vi "A170316-11_Auto.vi"() -> ()   [LabVIEW 2020]
uses:
  2e0b5f5e-2208-4490-a798-25a802626be8.vi
  Global_Variable/A170316-11.vi
  Global_Variable/Global.vi
  Database/Global1.vi
  <vilib>/addons/database/Connection.llb/DB Tools Open Connec (String).vi
  <vilib>/addons/database/NI_Database_API.lvlib
panel:
  out "电机安装螺栓2扭矩确认":bool
  out "请拾取O型圈":bool
  out "请拾取弹簧":bool
  in  "控制器支架":T1(ring)
  in  "ECU步骤":T2(ring)
  in  "电机步骤":T3(ring)
  out "产品型号":string
  in  "更换产品":refnum<vi>
  in  "前序OK？_ECU":string
  in  "前序OK？":string
  in  "Process":string[](array[string])
  in  "Code":string[](array[string])
  in  "User":string[](array[string])
  in  "Result":string[](array[string])
  in  "Device":string[](array[string])
  out "安装支架螺栓4拧紧确认":bool
  in  "STEP2":string
  in  "STEP1":string
  out "控制器安装螺栓3拧紧确认":bool
  out "电机安装螺栓1扭矩确认":bool
  out "控制器支架螺栓5拧紧确认":bool
  out "安装扎带并取走工件":bool
  out "涂色标":bool
  out "按启动按钮拍照确认":bool
  out "电机预拧紧螺栓2":bool
  out "电机预拧紧螺栓1":bool
  out "安装支架涂色标":bool
  out "控制器安装螺栓2拧紧确认":bool
  out "控制器安装螺栓1拧紧确认":bool
  out "安装支架螺栓2拧紧确认":bool
  out "安装弹性垫圈并按启动拍照":bool
  out "安装支架螺栓1拧紧确认":bool
  out "控制器支架涂色标":bool
  out "控制器支架螺栓4拧紧确认":bool
  out "控制器支架螺栓3拧紧确认":bool
  out "控制器支架螺栓2拧紧确认":bool
  out "控制器支架螺栓1拧紧确认":bool
  out "安装支架螺栓3拧紧确认":bool
  in  "更换布局":string
  out "安装扎带和线卡并取走工件":bool
  out "安装支架扎带安装":bool
  out "安装支架线卡扎带安装":bool
  out "控制器支架安装线卡扎带":bool
  out "磨合次数":i32
  in  "判定结果":bool[][](array[boolean])=[[TRUE]]
  in  "STEP3":string
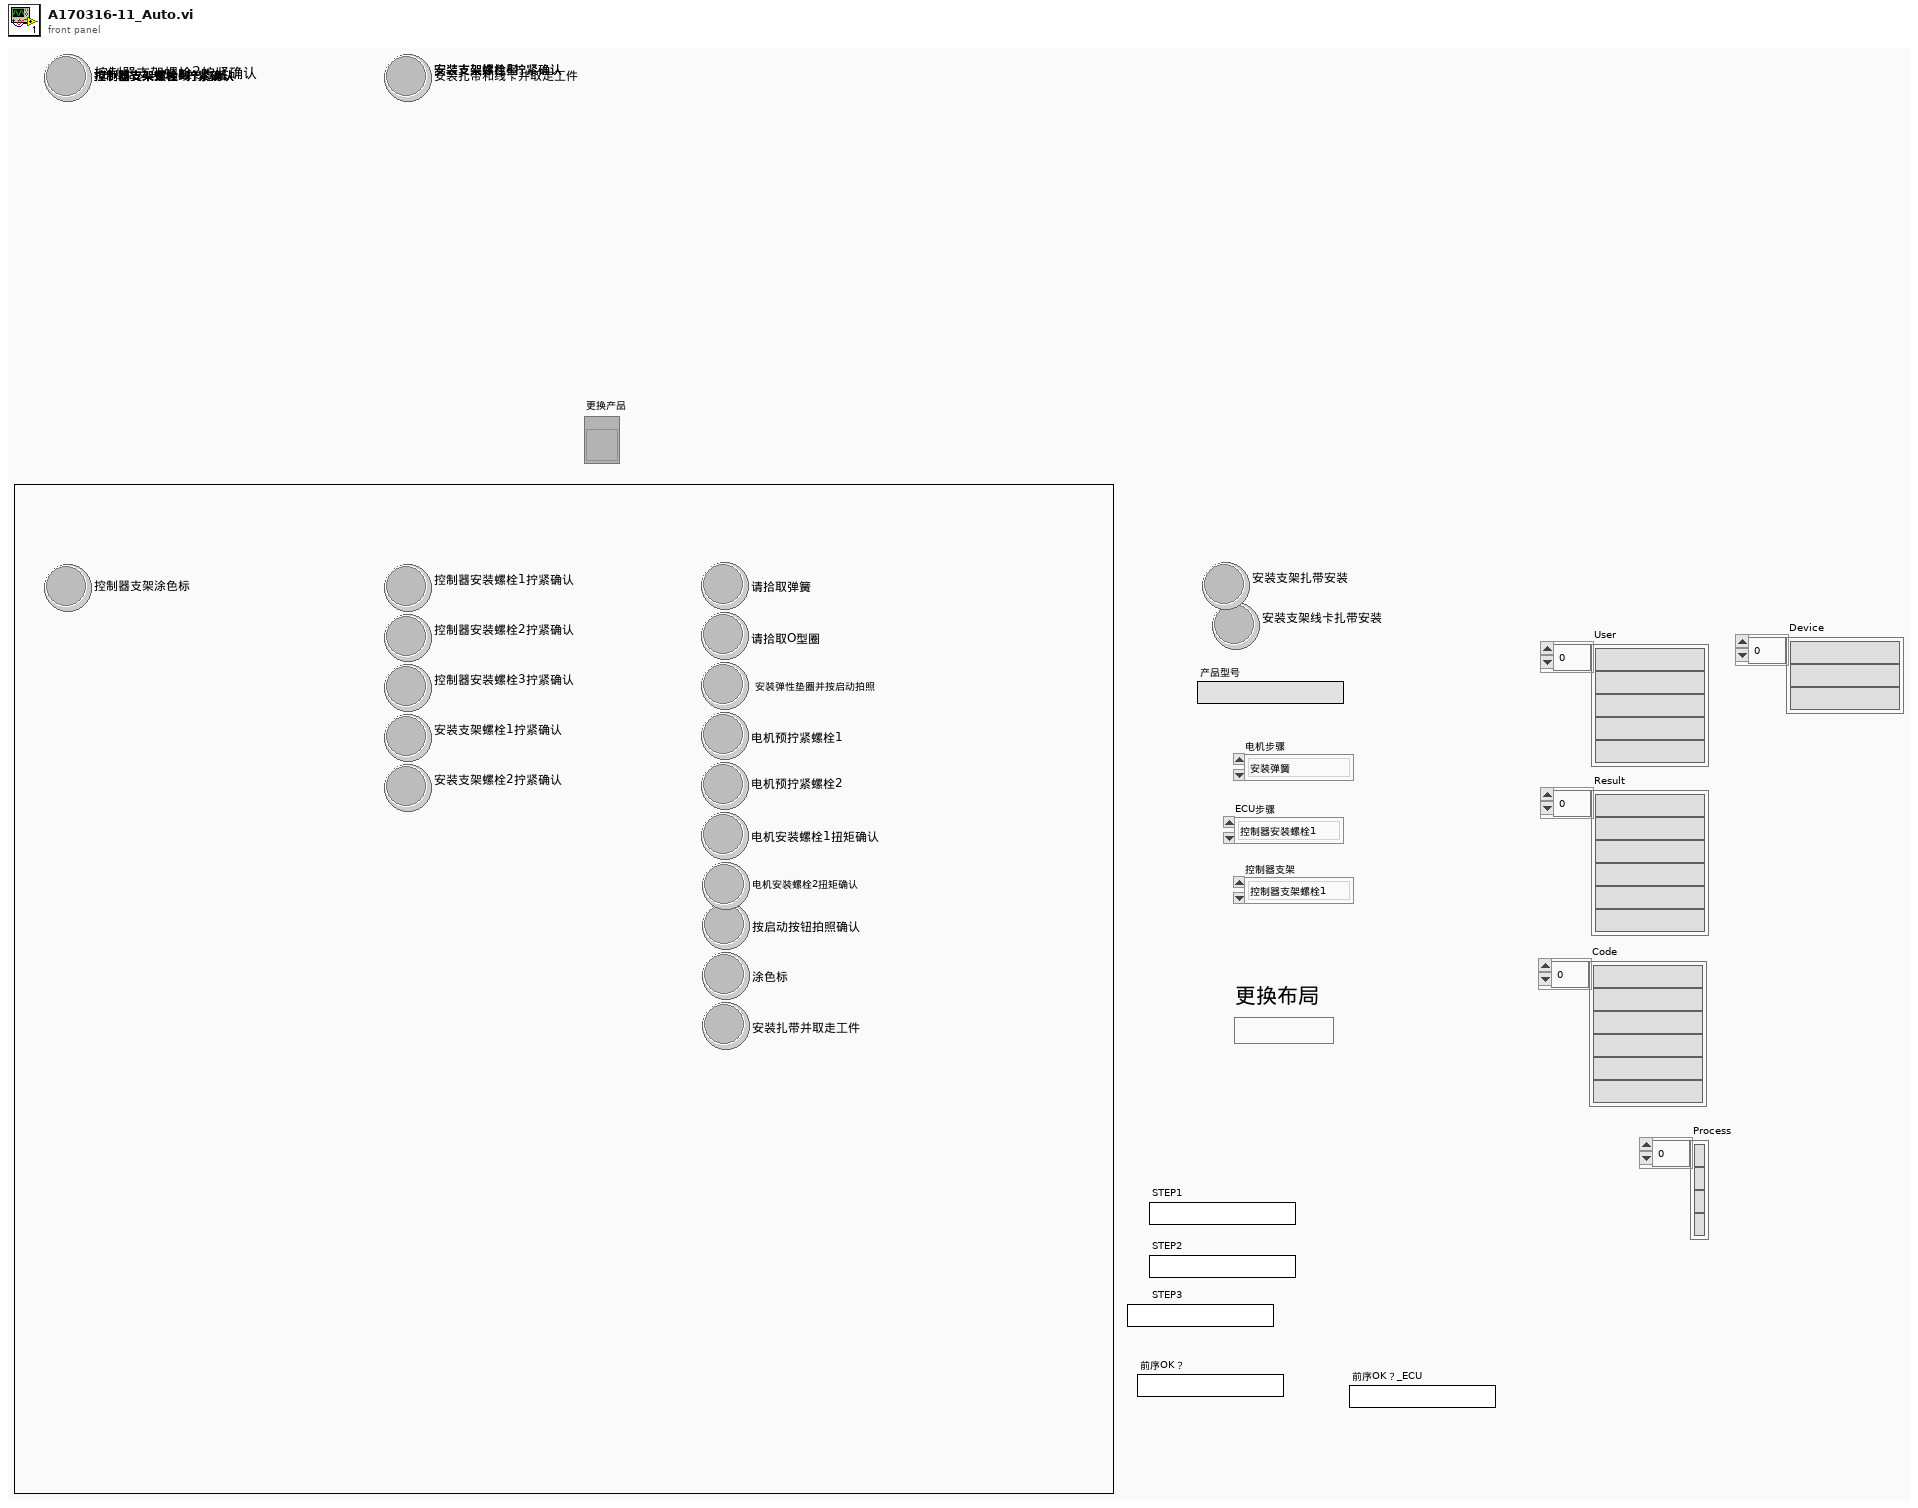
[diagram p1: front panel]
types:
  T1 = enum16{"控制器支架螺栓1", "控制器支架螺栓2", "控制器支架螺栓3", "控制器支架螺栓4", "控制器支架螺栓5", "涂色标", "安装线卡轧带", "完成"}
  T2 = enum16{"控制器安装螺栓1", "控制器安装螺栓2", "控制器安装螺栓3", "安装支架螺栓1", "安装支架螺栓2", "安装支架螺栓3", "安装支架螺栓4", "涂色标", "安装线卡取走工件", "完成"}
  T3 = enum16{"安装弹簧", "安装O型圈", "安装弹性垫圈", "预拧紧1", "预拧紧2", "电机1", "电机2", "电机拍照", "涂色标", "安装轧带取走工件", "完成"}
  T4 = cluster{i64, i64, i64, "电机工位生产结果":string, "result string":string}
  T5 = cluster{i64, i64, i64, "电机工位生产结果":string, "result string":string}[]
  T6 = typedef "NI_Database_API.lvlib/Conn ObjectReference.ctl" = refnum<k1>
  T7 = cluster{"电机工位生产结果":string, "result string":string}
  T8 = cluster{i64, i64, i64, "ECU工位生产结果":string, "result string":string}
  T9 = cluster{i64, i64, i64, "ECU工位生产结果":string, "result string":string}[]
  T10 = cluster{"ECU工位生产结果":string, "result string":string}
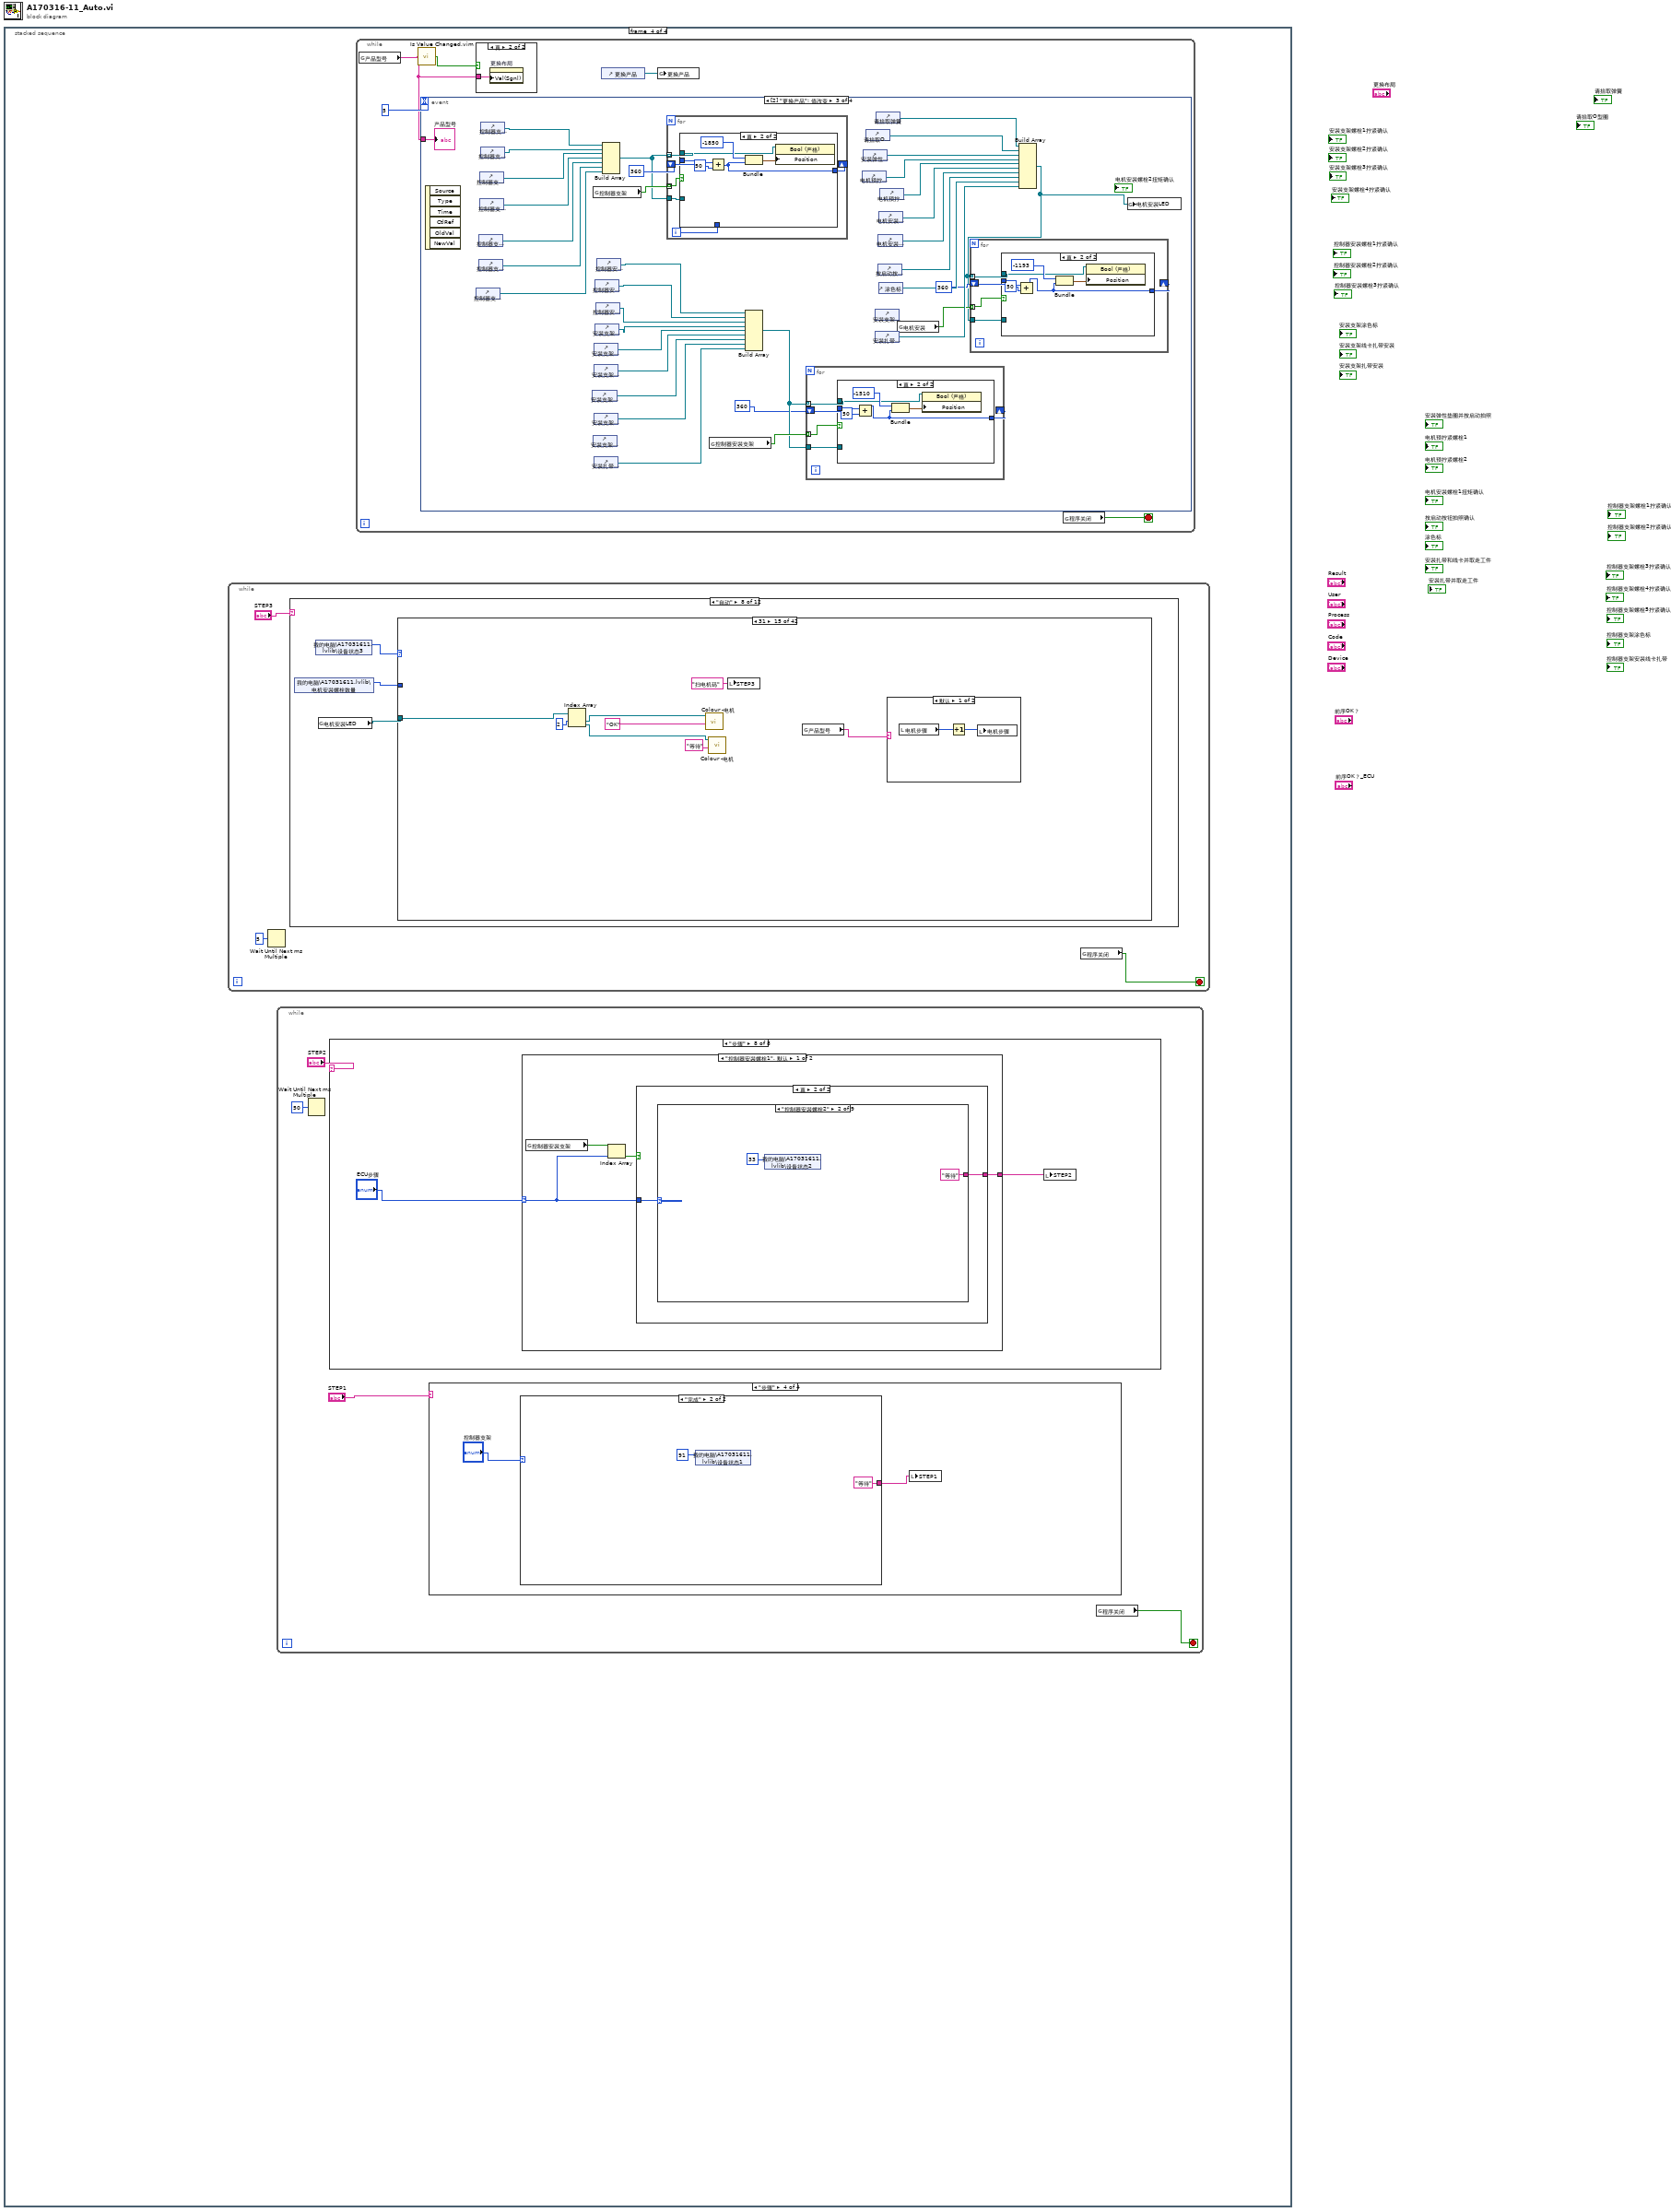
[diagram p0: block diagram]
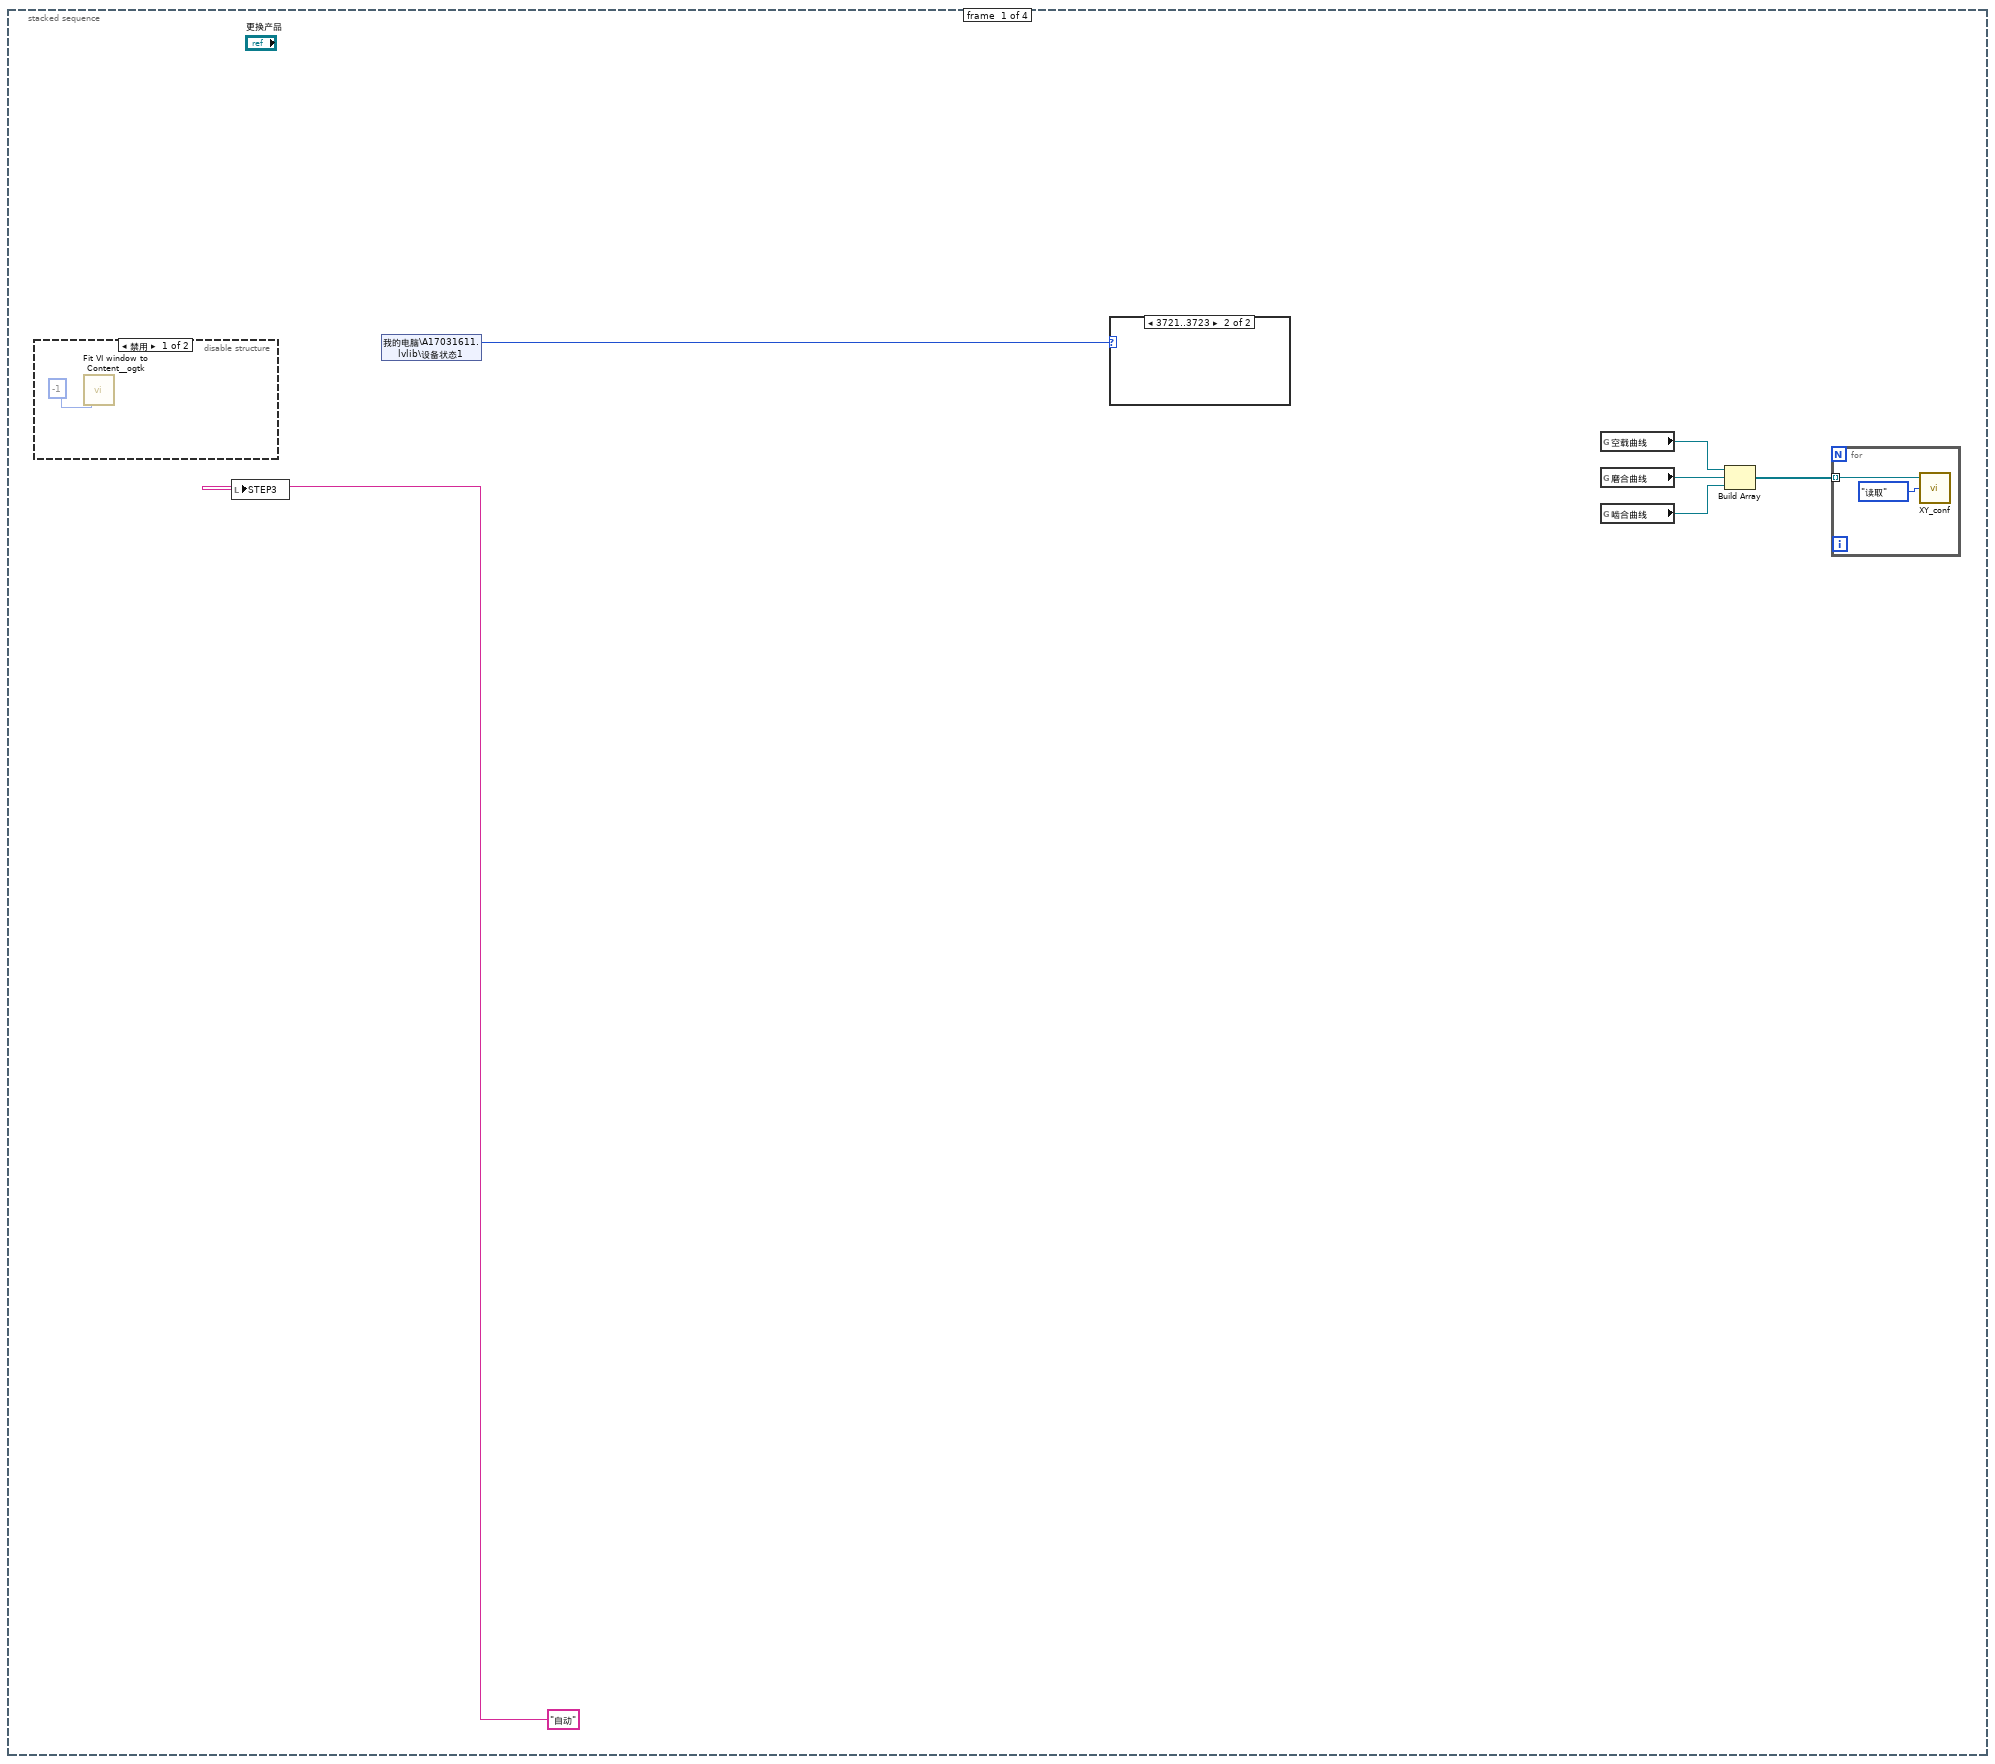
[diagram p2: hidden frame]
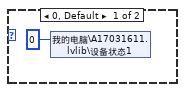
[diagram p4: hidden frame]
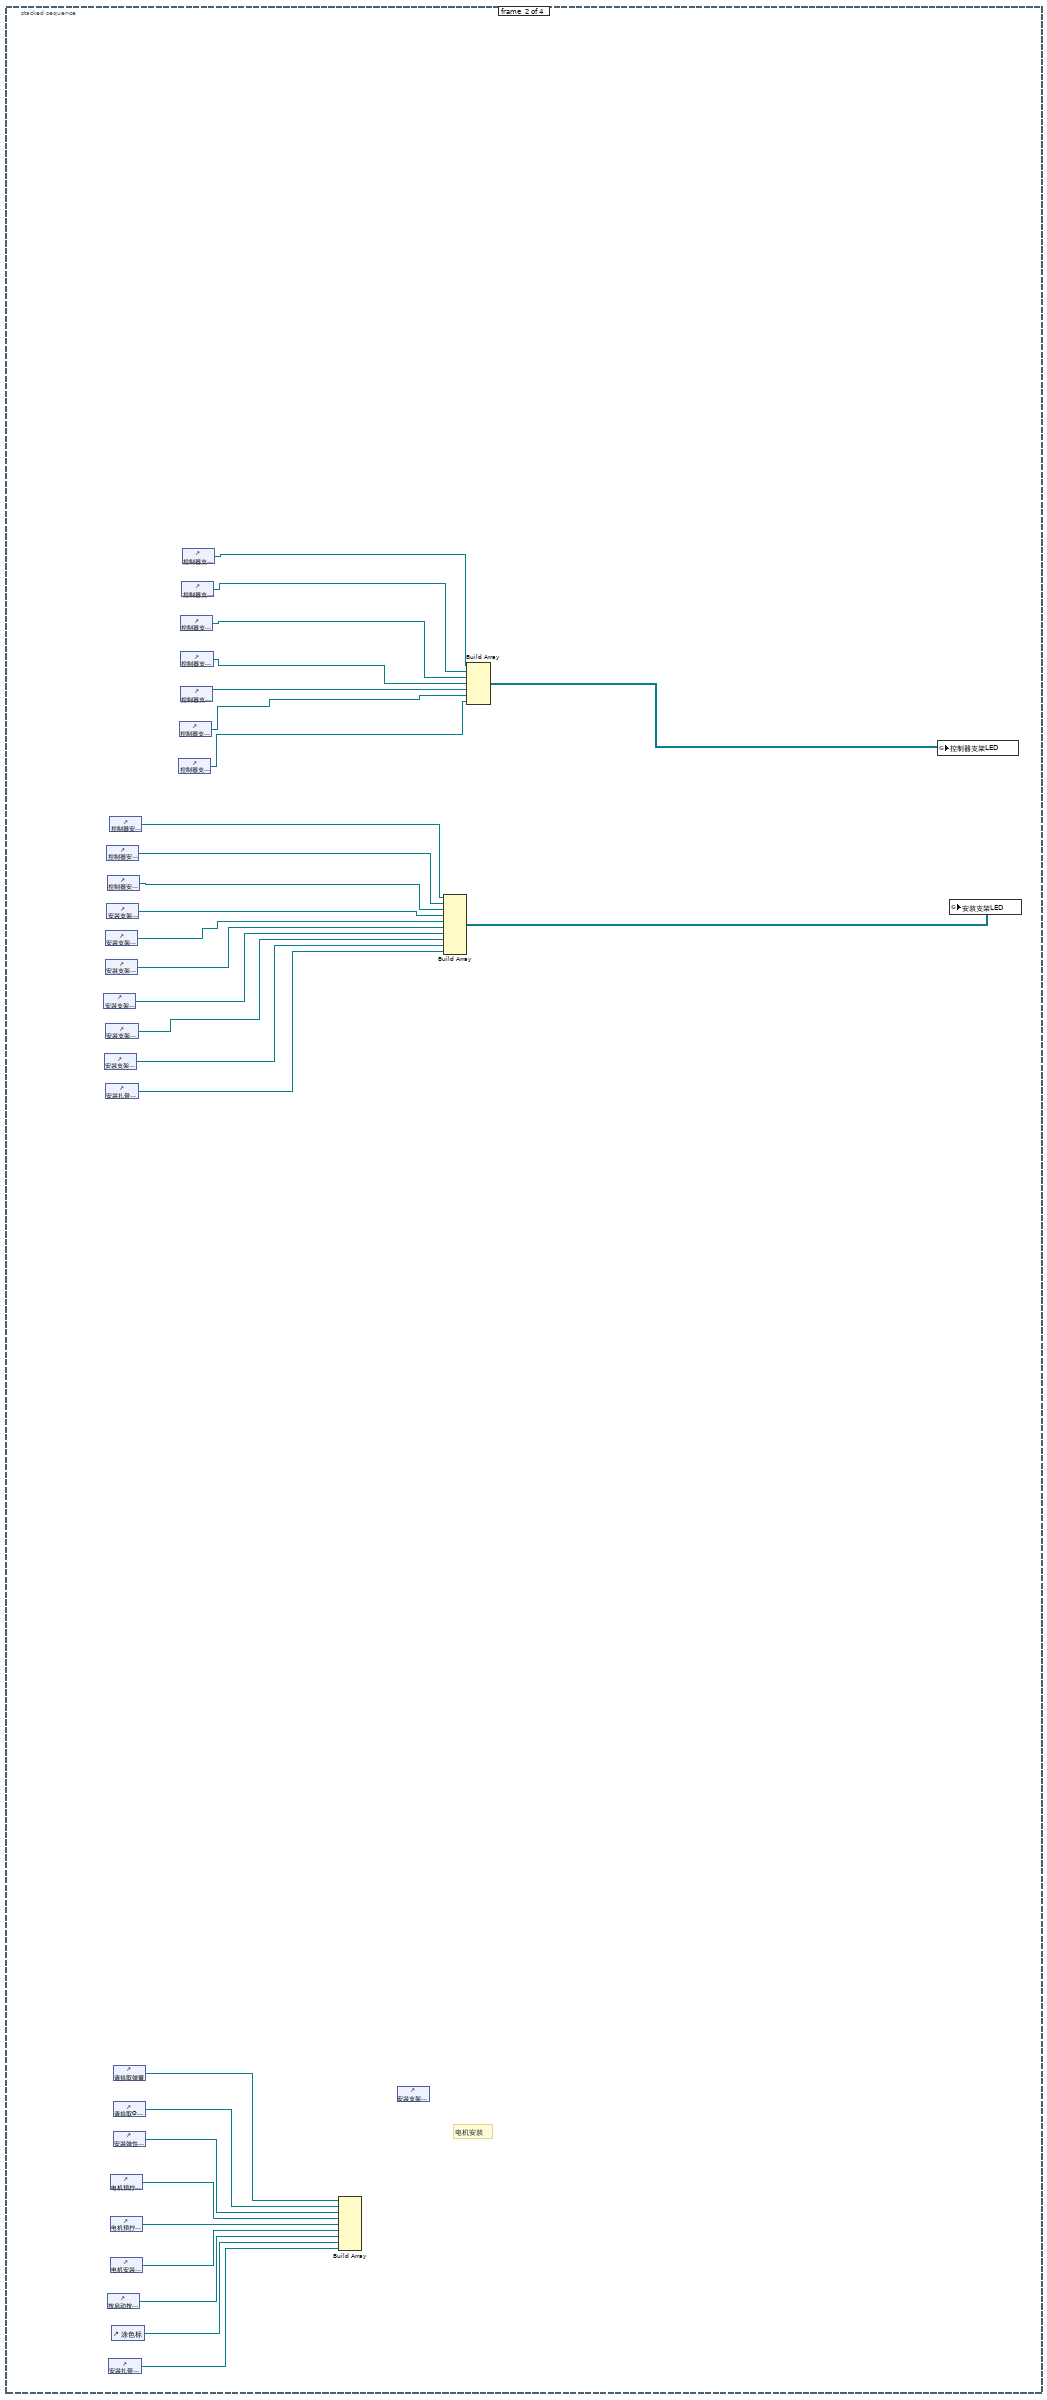
[diagram p5: hidden frame]
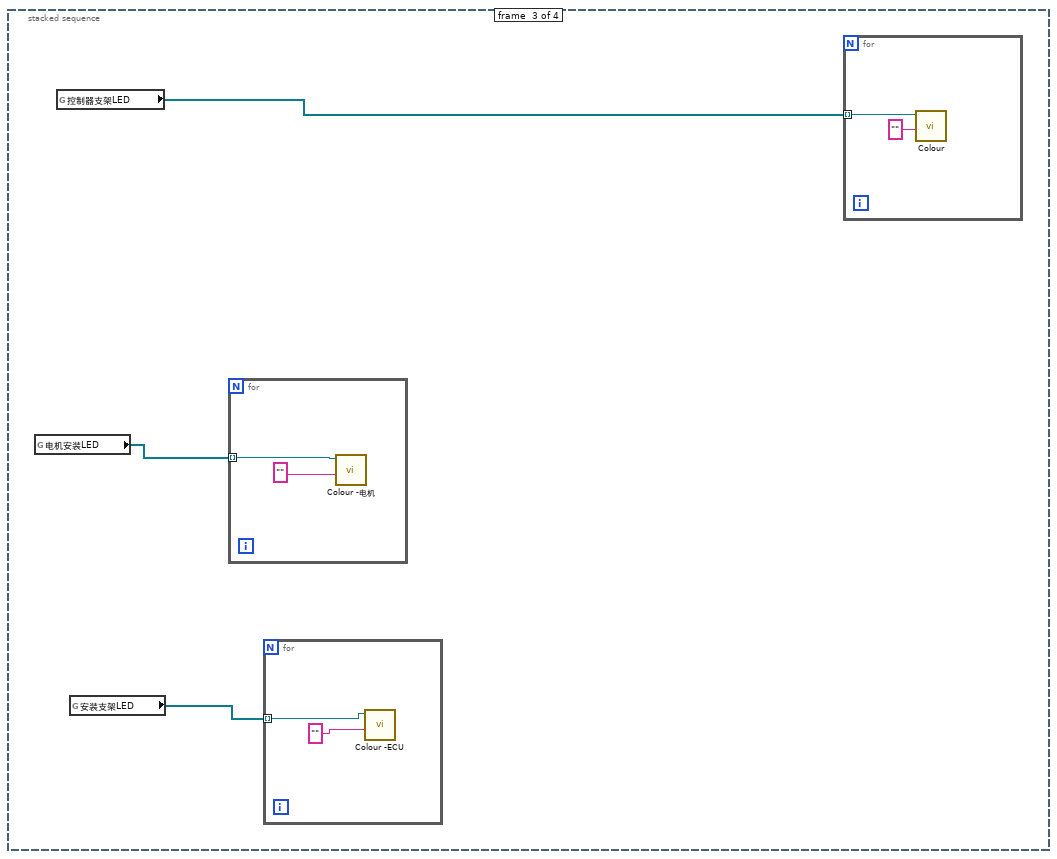
[diagram p6: hidden frame]
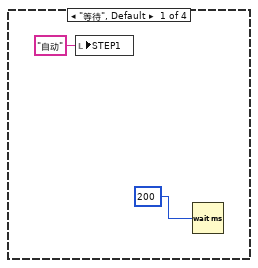
[diagram p7: hidden frame]
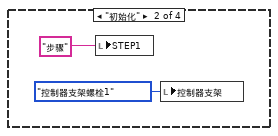
[diagram p8: hidden frame]
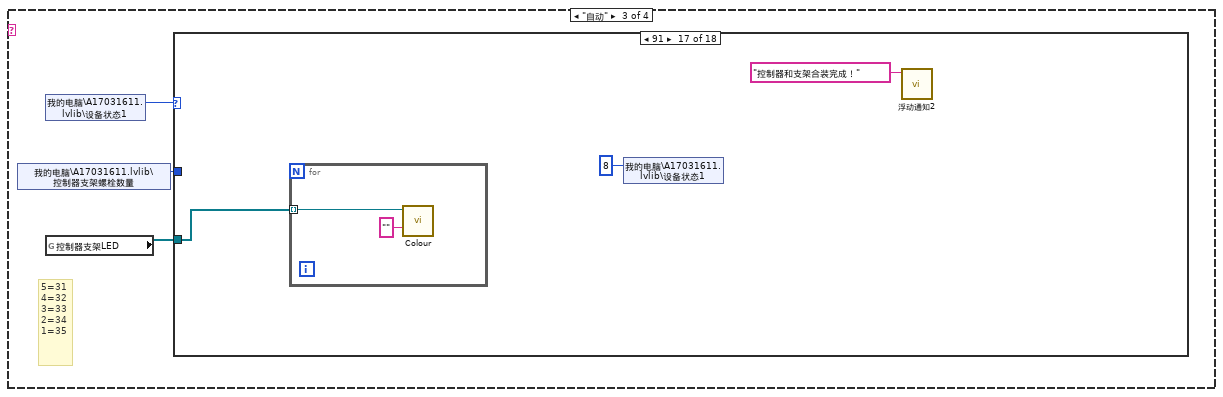
[diagram p9: hidden frame]
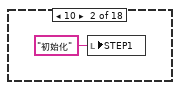
[diagram p11: hidden frame]
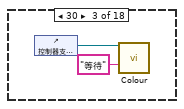
[diagram p12: hidden frame]
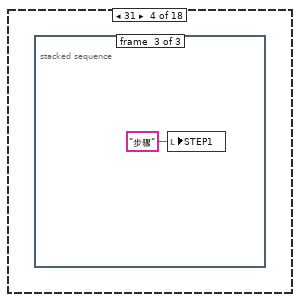
[diagram p13: hidden frame]
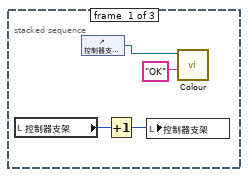
[diagram p14: hidden frame]
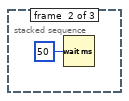
[diagram p15: hidden frame]
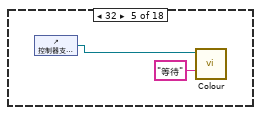
[diagram p16: hidden frame]
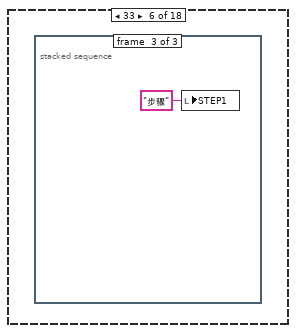
[diagram p17: hidden frame]
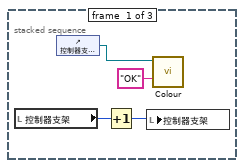
[diagram p18: hidden frame]
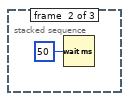
[diagram p19: hidden frame]
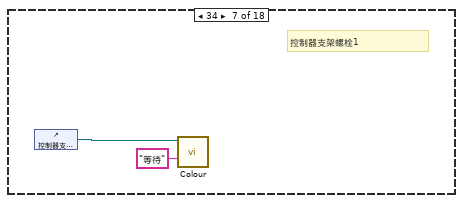
[diagram p20: hidden frame]
diagram:
  n1 = stacked-sequence {
    frame #0 {
      n2 = disable-structure shown="禁用" {
        frame Disabled {
          n3 = call "Fit VI window to Content__ogtk.vi"("border spacing (2 px)"=-1) -> ()  [unwired: 5 in, 2 out]
        }
        frame Enabled {
        }
      }
      n4 = local write "STEP3"("自动" ("STEP")) -> ()
      n5 = shared-variable "我的电脑\\A17031611.lvlib\\设备状态1"() -> (w4:i16)  [unwired: 1 in, 1 out]
      n6 = case shown="3721..3723" w4 {
        frame 0, Default {
          n7 = shared-variable "我的电脑\\A17031611.lvlib\\设备状态1"(i16 0 ("设备状态")) -> ()  [unwired: 1 in, 1 out]
        }
        frame 3721..3723 {
        }
      }
      n8 = global read "A170316-11.vi" "空载曲线"() -> (w1:refnum<vi>)
      n9 = global read "A170316-11.vi" "磨合曲线"() -> (w2:refnum<vi>)
      n10 = global read "A170316-11.vi" "啮合曲线"() -> (w3:refnum<vi>)
      n11 = Build Array(w1, w2, w3) -> (w5:refnum<vi>[])
      n12 = for {
        tunnel: w5 -> [w10] mode=indexing
        n13 = call "XY_conf.vi"("方式"=enum16{"写入", "读取"}."读取", "XY图引用"=w10) -> ()  [unwired: 3 in, 1 out]
      }
    }
    frame #1 {
      # "电机安装"
      n14 = control-ref of="安装支架螺栓4拧紧确认"() -> (w16:refnum<vi>)
      n15 = control-ref of="安装支架线卡扎带安装"() -> (w14:refnum<vi>)
      n16 = control-ref of="安装支架螺栓2拧紧确认"() -> (w18:refnum<vi>)
      n17 = control-ref of="安装支架螺栓3拧紧确认"() -> (w17:refnum<vi>)
      n18 = control-ref of="安装支架涂色标"() -> (w15:refnum<vi>)
      n19 = control-ref of="安装扎带和线卡并取走工件"() -> (w13:refnum<vi>)
      n20 = control-ref of="控制器安装螺栓2拧紧确认"() -> (w21:refnum<vi>)
      n21 = control-ref of="安装支架螺栓1拧紧确认"() -> (w19:refnum<vi>)
      n22 = control-ref of="控制器安装螺栓3拧紧确认"() -> (w20:refnum<vi>)
      n23 = control-ref of="按启动按钮拍照确认"() -> (w25:refnum<vi>)
      n24 = control-ref of="安装扎带并取走工件"() -> (w23:refnum<vi>)
      n25 = control-ref of="控制器安装螺栓1拧紧确认"() -> (w22:refnum<vi>)
      n26 = control-ref of="电机预拧紧螺栓1"() -> (w28:refnum<vi>)
      n27 = control-ref of="电机预拧紧螺栓2"() -> (w27:refnum<vi>)
      n28 = control-ref of="电机安装螺栓1扭矩确认"() -> (w26:refnum<vi>)
      n29 = control-ref of="涂色标"() -> (w24:refnum<vi>)
      n30 = control-ref of="请拾取弹簧"() -> (w12:refnum<vi>)
      n31 = control-ref of="请拾取O型圈"() -> (w11:refnum<vi>)
      n32 = control-ref of="安装弹性垫圈并按启动拍照"() -> (w29:refnum<vi>)
      n33 = control-ref of="控制器支架安装线卡扎带"() -> (w30:refnum<vi>)
      n34 = control-ref of="控制器支架涂色标"() -> (w31:refnum<vi>)
      n35 = control-ref of="控制器支架螺栓3拧紧确认"() -> (w34:refnum<vi>)
      n36 = control-ref of="控制器支架螺栓5拧紧确认"() -> (w32:refnum<vi>)
      n37 = control-ref of="控制器支架螺栓4拧紧确认"() -> (w33:refnum<vi>)
      n38 = control-ref of="控制器支架螺栓2拧紧确认"() -> (w35:refnum<vi>)
      n39 = control-ref of="控制器支架螺栓1拧紧确认"() -> (w36:refnum<vi>)
      n40 = Build Array(w12, w11, w29, w28, w27, w26, w25, w24, w23) -> ()  [unwired: 1 out]
      n41 = control-ref of="安装支架扎带安装"() -> ()  [unwired: 1 out]
      n42 = Build Array(w22, w21, w20, w19, w18, w17, w16, w15, w14, w13) -> (w38:refnum<vi>[])
      n43 = Build Array(w36, w35, w34, w33, w32, w31, w30) -> (w37:refnum<vi>[])
      n44 = global write "A170316-11.vi" "控制器支架LED"(w37) -> ()
      n45 = global write "A170316-11.vi" "安装支架LED"(w38) -> ()
    }
    frame #2 {
      n46 = global read "A170316-11.vi" "电机安装LED"() -> (w40:refnum<vi>[])
      n47 = global read "A170316-11.vi" "控制器支架LED"() -> (w41:refnum<vi>[])
      n48 = global read "A170316-11.vi" "安装支架LED"() -> (w39:refnum<vi>[])
      n49 = for {
        tunnel: w40 -> [w45] mode=indexing
        n50 = call "Colour -电机.vi"("result"="", "colourRef"=w45) -> ()  [unwired: 9 in, 1 out]
      }
      n51 = for {
        tunnel: w39 -> [w43] mode=indexing
        n52 = call "Colour -ECU.vi"("result"="", "colourRef"=w43) -> ()  [unwired: 9 in, 1 out]
      }
      n53 = for {
        tunnel: w41 -> [w46] mode=indexing
        n54 = call "Colour.vi"("result"="", "colourRef"=w46) -> ()  [unwired: 9 in, 1 out]
      }
    }
    frame #3 {
      n55 = while {
        stop <- w550 stop-if-true
        n56 = Wait Until Next ms Multiple(millisecond multiple=u32 5 ("等待时间（毫秒）")) -> ()  [unwired: 1 out]
        n57 = case shown="\"自动\"" "STEP3" {
          frame "等待", Default {
            n58 = local write "STEP3"("自动" ("STEP")) -> ()
            n59 = Wait (ms)(milliseconds to wait=u32 100 ("等待时间（毫秒）")) -> ()  [unwired: 1 out]
          }
          frame "手动" {
          }
          frame "初始化" {
            n60 = stacked-sequence {
              frame #0 {
                w563 = enum16{"录入", "清空"}."清空" ("功能")
                n61 = global read "Global.vi" "电机生产数量"() -> (w556:refnum<vi>)
                n62 = shared-variable "我的电脑\\Global.lvlib\\工位追溯码"("" ("传感器码")) -> ()  [unwired: 1 in, 1 out]
                n63 = call "物料信息录入.vi"("功能"=w563) -> ("错误输出"=w562:errorcluster)  [unwired: 14 in]
                n64 = call "质量信息录入.vi"("功能"=w563, "错误输入（无错误）"=w562) -> ("错误输出"=w564:errorcluster)  [unwired: 13 in]
                n65 = property class="Num"(reference=w556, "Value"=0 ("磨合次数")) -> ()  [unwired: 1 in, 2 out]
                n66 = call "不合格信息录入.vi"("功能"=w563, "错误输入（无错误）"=w564) -> ()  [unwired: 13 in, 1 out]
                n67 = global read "Global.vi" "电机程序自动"() -> (w560:refnum<vi>)
                n68 = global read "Global.vi" "检测结果"() -> (w558:refnum<vi>)
                n69 = shared-variable "我的电脑\\A17031611.lvlib\\设备状态3"(i16 6 ("设备状态")) -> ()  [unwired: 1 in, 1 out]
                n70 = property class="Bool"(reference=w560, "Value"=TRUE) -> ()  [unwired: 1 in, 2 out]
                n71 = call "Colour.vi"("result"="", "colourRef"=w558) -> ()  [unwired: 9 in, 1 out]
              }
              frame #1 {
                n72 = for {
                  N: 2 -> [_]
                  tunnel: [cluster{dbl[], dbl[]} {[], []}] -> _ mode=indexing
                }
              }
              frame #2 {
                n73 = global read "Global.vi" "Result"() -> (w569:refnum<vi>)
                n74 = property class="Tbl"(reference=w569, "Value"=string[][] []) -> (reference out=w570:refnum<vi>, error out=w571:errorcluster)  [unwired: 1 in]
                n75 = property class="Tbl"(reference=w570, error in=w571, "Row Headers[]"=string[] ["正向空载扭矩最大值", "正向空载扭矩最小值", "正向空载扭矩平均值", "正向空载扭矩波动值", "逆向空载扭矩最大值", "逆向空载扭矩最小值", "逆向空载扭矩平均值", "逆向空载扭矩波动值", "啮合间隙"] ("列首字符串[]")) -> ()  [unwired: 2 out]
              }
              frame #3 {
                n76 = local write "电机步骤"(T3."安装弹簧" ("电机步骤")) -> ()
                n77 = local write "STEP3"("等待" ("STEP")) -> ()
              }
            }
          }
          frame "批次数量判断" {
            n78 = shared-variable "我的电脑\\Global.lvlib\\产品型号"() -> (w579:string, error out=w582:errorcluster)  [unwired: 1 in]
            n79 = global read "Global.vi" "批次"() -> (w580:refnum<vi>)
            n80 = call "获取批次信息.vi"("error in (no error)"=w582, "产品型号"=w579, "Tbl引用句柄"=w580) -> ("error out"=w581:errorcluster)  [unwired: 7 in, 1 out]
            n81 = property class="Tbl"(reference=w580, error in=w581) -> ("Value"=w583:string[][])  [unwired: 2 out]
            n82 = for {
              tunnel: w583 -> [w589] mode=indexing
              tunnel: [w584] -> w578 mode=indexing
              n83 = Index Array(array=w589) -> (element #1=w585:string, element #3=w588:string)  [unwired: 3 in, 1 out]
              n84 = Decimal String To Number(string=w588) -> (number=w587:i32)  [unwired: 2 in, 1 out]
              n85 = Less Or Equal To 0?(x=w587) -> (x <= 0?=w586:bool)
              n86 = case shown="真" w586 {
                tunnel: w585 -> [_ w594]
                tunnel: [TRUE FALSE] -> w584
                frame False {
                }
                frame True {
                  n87 = Concatenate Strings(w594, "数量不足！" ("字符串")) -> (w592:string)
                  n88 = One Button Dialog(message=w592) -> ()  [unwired: 1 in, 1 out]
                }
              }
            }
            n89 = And Array Elements(Boolean array=w578) -> (logical AND=w577:bool)
            n90 = Select(t="扫码" ("STEP"), s=w577, f="手动" ("STEP")) -> (s? t:f=w574:string)
            n91 = local write "STEP3"(w574) -> ()
          }
          frame "扫管柱码" {
            n92 = stacked-sequence {
              frame #0 {
                (unwired) "SELECT\ndbo.[Code].CODE_ID,\ndbo.[Code].CODE_MAIN,\ndbo.[Code].PRODUCT_ID\n\nFROM\ndbo.[Code].CODE_MAIN = 'MACAU3001'" ("格式字符串")
                (unwired) "SELECT\n*\nFROM\ndbo.[Code]\nWHERE\ndbo.[Code].CODE_MAIN = 'MACAU3001'" ("格式字符串")
                (unwired) "UPDATE\ndbo.[Code]\nSET dbo.[Code].CODE_SENSOR = 'henglong'\nWHERE\ndbo.[Code].CODE_MAIN = 'MACAU3001'\n" ("格式字符串")
                w595 = "请扫电机工位主码！" ("提示信息")
                n93 = global read "Global1.vi" "联机模式"() -> (w597:enum16{"单机", "联网"})
                n94 = call "输入框.vi"("提示信息"=w595) -> ("条形码输出"=w596:string)
                n95 = global write "Global1.vi" "电机工位追溯码"(w596) -> ()
                n96 = shared-variable "我的电脑\\Global.lvlib\\工位追溯码"(w596) -> ()  [unwired: 1 in, 1 out]
                n97 = call "浮动通知.vi"("通知内容"=w595) -> ()  [unwired: 11 in]
                n98 = case shown="\"\", 默认" w596 {
                  selector: w596 -> [w601 _]
                  tunnel: [w600 "手动"] -> w598
                  tunnel: w597 -> [w599 _]
                  frame "", Default {
                    n99 = case shown="\"联网\"" w599 {
                      tunnel: w601 -> [_ w611]
                      tunnel: ["步骤" ("State(s) in Front (\"\")") w610] -> w600
                      frame "单机", Default {
                        n100 = global read "Global.vi" "电机生产数量"() -> (w604:refnum<vi>)
                        n101 = property class="Num"(reference=w604) -> (reference out=w602:refnum<vi>, error out=w606:errorcluster, "Value"=w607:variant)  [unwired: 1 in]
                        n102 = Variant To Data(type=u32 0, Variant=w607) -> (data=w608:u32)  [unwired: 1 in, 1 out]
                        n103 = Increment(x=w608) -> (x+1=w609:u32)
                        n104 = property class="Num"(reference=w602, error in=w606, "Value"=w609) -> ()  [unwired: 2 out]
                      }
                      frame "联网" {
                        n105 = stacked-sequence {
                          tunnel: w611 -> [w618 _ _ _]
                          tunnel: [_ _ _ w640] -> w610
                          frame #0 {
                            n106 = global read "Global1.vi" "PRODUCT_ID"() -> (w615:string)
                            n107 = Format Into String(format string="SELECT\ndbo.[Code].CODE_ID\nFROM\ndbo.[Code]\nWHERE\ndbo.[Code].CODE_MAIN = '%s'\nAND\ndbo.[Code].PRODUCT_ID = %s\n" ("格式字符串"), w618, w615) -> (resulting string=w617:string)  [unwired: 2 in, 1 out]
                            n108 = call "SQL_query.vi"("SQL query"=w617, "联机模式"=enum16{"单机", "联网"}."联网") -> ("data"=w621:string[][])  [unwired: 1 in, 2 out]
                            n109 = Index Array(array=w621, index (row)=0 ("索引 (行)")) -> (element=w620:string[])  [unwired: 1 in]
                            n110 = Index Array(array=w620, index=0 ("索引")) -> (element=w612:string)
                            n111 = global write "Global1.vi" "CODE_ID"(w612) -> ()
                          }
                          frame #1 {
                            n112 = global read "Global1.vi" "前序DEVICE_ID"() -> (w622:string)
                            n113 = global read "Global1.vi" "CODE_ID"() -> (w623:string)
                            n114 = Format Into String(format string="SELECT\ndbo.[Result].RESULT_VALUE\nFROM\ndbo.[Result]\nWHERE\ndbo.[Result].DEVICE_ID = '%s'\nAND\ndbo.[Result].CODE_ID = %s\n" ("格式字符串"), w622, w623) -> (resulting string=w628:string)  [unwired: 2 in, 1 out]
                            n115 = call "SQL_query.vi"("SQL query"=w628, "联机模式"=enum16{"单机", "联网"}."联网") -> ("data"=w631:string[][])  [unwired: 1 in, 2 out]
                            n116 = Index Array(array=w631, index (row)=0 ("索引 (行)")) -> (element=w630:string[])  [unwired: 1 in]
                            n117 = Index Array(array=w630, index=0 ("索引")) -> (element=w624:string)
                            n118 = local write "前序OK？"(w624) -> ()
                          }
                          frame #2 {
                            n119 = disable-structure shown="禁用" {
                              frame Disabled {
                                n120 = global read "Global1.vi" "CODE_ID"() -> (w633:string)
                                n121 = Format Into String(format string="SELECT\ndbo.[Result].RESULT_VALUE\nFROM\ndbo.[Result]\nWHERE\ndbo.[Result].CODE_ID = '%s''" ("格式字符串"), w633) -> (resulting string=w635:string)  [unwired: 2 in, 1 out]
                                n122 = call "SQL_query.vi"("SQL query"=w635, "联机模式"=enum16{"单机", "联网"}."联网") -> ("data"=w638:string[][])  [unwired: 1 in, 2 out]
                                n123 = Index Array(array=w638) -> (element=w636:string[])  [unwired: 2 in]
                                n124 = Index Array(array=w636) -> (element=w637:string)  [unwired: 1 in]
                                n125 = global write "Global1.vi" "RESULT_VALUE"(w637) -> ()
                              }
                              frame Enabled {
                              }
                            }
                          }
                          frame #3 {
                            n126 = local read "前序OK？"() -> (w639:string)
                            n127 = case shown="\"OK\"" w639 {
                              tunnel: ["自动" "自动" "步骤"] -> w640
                              tunnel: [i16 6 ("设备状态3") u32 6 ("等待时间（毫秒）") u32 16 ("等待时间（毫秒）")] -> _
                              frame Default {
                                n128 = global read "Global1.vi" "电机上序状态"() -> (w646:refnum<vi>)
                                n129 = call "浮动通知.vi"("通知内容"="上序漏序！！" ("Status")) -> ()  [unwired: 11 in]
                                n130 = global read "Global.vi" "电机前序显示字"() -> (w644:refnum<vi>)
                                n131 = call "Colour.vi"("result"="等待", "colourRef"=w646) -> ()  [unwired: 9 in, 1 out]
                                n132 = Wait (ms)(milliseconds to wait=u32 2000 ("等待时间（毫秒）")) -> ()  [unwired: 1 out]
                                n133 = property class="Str"(reference=w644, "Value"="漏序 " ("值")) -> ()  [unwired: 1 in, 2 out]
                              }
                              frame "NG" {
                                n134 = global read "Global1.vi" "电机上序状态"() -> (w653:refnum<vi>)
                                n135 = call "浮动通知.vi"("通知内容"="上序生产结果不合格！" ("Status")) -> ()  [unwired: 11 in]
                                n136 = global read "Global.vi" "电机前序显示字"() -> (w651:refnum<vi>)
                                n137 = call "Colour.vi"("result"="NG", "colourRef"=w653) -> ()  [unwired: 9 in, 1 out]
                                n138 = Wait (ms)(milliseconds to wait=u32 2000 ("等待时间（毫秒）")) -> ()  [unwired: 1 out]
                                n139 = property class="Str"(reference=w651, "Value"="NG " ("值")) -> ()  [unwired: 1 in, 2 out]
                              }
                              frame "OK" {
                                n140 = global read "Global.vi" "电机生产数量"() -> (w669:refnum<vi>)
                                n141 = global read "Global1.vi" "电机上序状态"() -> (w662:refnum<vi>)
                                n142 = property class="Num"(reference=w669) -> (reference out=w670:refnum<vi>, error out=w668:errorcluster, "Value"=w667:variant)  [unwired: 1 in]
                                n143 = global read "Global.vi" "电机前序显示字"() -> (w660:refnum<vi>)
                                n144 = call "Colour.vi"("result"="OK", "colourRef"=w662) -> ()  [unwired: 9 in, 1 out]
                                n145 = Variant To Data(type=u32 0, Variant=w667) -> (data=w666:u32)  [unwired: 1 in, 1 out]
                                n146 = Increment(x=w666) -> (x+1=w665:u32)
                                n147 = property class="Num"(reference=w670, error in=w668, "Value"=w665) -> ()  [unwired: 2 out]
                                n148 = property class="Str"(reference=w660, "Value"="OK" ("值")) -> ()  [unwired: 1 in, 2 out]
                                n149 = Wait (ms)(milliseconds to wait=u32 1000 ("等待时间（毫秒）")) -> ()  [unwired: 1 out]
                              }
                            }
                          }
                        }
                      }
                    }
                  }
                  frame "exit" {
                  }
                }
                n150 = local write "STEP3"(w598) -> ()
              }
              frame #1 {
                n151 = Wait (ms)(milliseconds to wait=u32 200 ("等待时间（毫秒）")) -> ()  [unwired: 1 out]
              }
            }
          }
          frame "扫电机码" {
            n152 = stacked-sequence {
              frame #0 {
                w673 = "请扫电机码！" ("提示信息")
                n153 = call "输入框.vi"("提示信息"=w673) -> ("条形码输出"=w674:string)
                n154 = call "浮动通知.vi"("通知内容"=w673) -> ()  [unwired: 11 in]
                n155 = case shown="\"\", 默认" w674 {
                  selector: w674 -> [w676 _]
                  tunnel: [w677 "手动"] -> w675
                  frame "", Default {
                    n156 = global read "Global1.vi" "联机模式"() -> (w678:enum16{"单机", "联网"})
                    n157 = shared-variable "我的电脑\\Global.lvlib\\电机码"(w676) -> ()  [unwired: 1 in, 1 out]
                    n158 = global write "Global1.vi" "电机码"(w676) -> ()
                    n159 = case shown="\"单机\", 默认" w678 {
                      tunnel: w676 -> [_ _]
                      tunnel: ["步骤" ("State(s) in Front (\"\")") "步骤" ("State(s) in Front (\"\")")] -> w677
                      frame "单机", Default {
                        n160 = shared-variable "我的电脑\\A17031611.lvlib\\设备状态3"(i16 0 ("设备状态控制字")) -> ()  [unwired: 1 in, 1 out]
                      }
                      frame "联网" {
                        n161 = disable-structure shown="禁用" {
                          frame Disabled {
                            n162 = shared-variable "我的电脑\\A17031611.lvlib\\电机安装螺栓数量"() -> (w683:i16)  [unwired: 1 in, 1 out]
                            n163 = case shown="2, 默认" w683 {
                              frame 2, Default {
                                n164 = shared-variable "我的电脑\\A17031611.lvlib\\设备状态3"(i16 41 ("设备状态控制字")) -> ()  [unwired: 1 in, 1 out]
                              }
                              frame 3 {
                                n165 = shared-variable "我的电脑\\A17031611.lvlib\\设备状态3"(i16 40 ("设备状态控制字")) -> ()  [unwired: 1 in, 1 out]
                              }
                            }
                          }
                          frame Enabled {
                          }
                        }
                        n166 = shared-variable "我的电脑\\A17031611.lvlib\\设备状态3"(i16 0 ("设备状态控制字")) -> ()  [unwired: 1 in, 1 out]
                      }
                    }
                  }
                  frame "exit" {
                  }
                }
                n167 = local write "STEP3"(w675) -> ()
              }
              frame #1 {
                n168 = Wait (ms)(milliseconds to wait=u32 100 ("等待时间（毫秒）")) -> ()  [unwired: 1 out]
              }
            }
          }
          frame "录入批次" {
            n169 = shared-variable "我的电脑\\Global.lvlib\\产品型号"() -> (w689:string)  [unwired: 1 in, 1 out]
            n170 = call "更新批次.vi"("型号"=w689) -> ("error out"=w690:errorcluster)  [unwired: 10 in]
            n171 = call "更新易损件.vi"("error in (no error)"=w690) -> ("error out"=w693:errorcluster)  [unwired: 10 in]
            n172 = global read "Global.vi" "批次"() -> (w691:refnum<vi>)
            n173 = property class="Tbl"(reference=w691, error in=w693) -> ("Value"=w692:string[][])  [unwired: 2 out]
            n174 = for {
              tunnel: w692 -> [w696] mode=indexing
              n175 = Index Array(array=w696) -> (element #1=w695:string, element #2=w694:string)  [unwired: 2 in]
              n176 = call "物料信息录入.vi"("物料名称"=w695, "功能"=enum16{"录入", "清空"}."录入", "物料编码"=w694) -> ()  [unwired: 12 in, 1 out]
            }
            n177 = local write "STEP3"("等待" ("STEP")) -> ()
          }
          frame "自动" {
            n178 = shared-variable "我的电脑\\A17031611.lvlib\\电机安装螺栓数量"() -> (w698:i16)  [unwired: 1 in, 1 out]
            n179 = shared-variable "我的电脑\\A17031611.lvlib\\设备状态3"() -> (w699:i16)  [unwired: 1 in, 1 out]
            n180 = global read "A170316-11.vi" "电机安装LED"() -> (w700:refnum<vi>[])
            n181 = case shown="31" w699 {
              tunnel: w698 -> [_ _ _ _ _ _ _ _ _ _ _ _ _ _ _ w762 w772 _ _ _ _ _ _ _ _ w846 w858 _ _ _ _ _ _ _ _ _ _ _ _ _ _ _]
              tunnel: w700 -> [_ _ _ _ w707 _ _ _ w722 w729 w732 w739 w743 w748 w757 w764 w771 w799 w807 w811 w819 w823 w831 w836 w843 w845 w857 w869 w875 w882 w886 w894 w898 w904 _ _ w934 _ _ _ _ _]
              frame -128 {
                n182 = call "浮动通知.vi"("通知内容"="复位中……" ("Status")) -> ()  [unwired: 11 in]
                n183 = global read "Global.vi" "电机程序自动"() -> (w702:refnum<vi>)
                n184 = property class="Bool"(reference=w702, "Value"=FALSE) -> ()  [unwired: 1 in, 2 out]
              }
              frame 0 {
              }
              frame 5 {
                n185 = call "浮动通知.vi"("通知内容"="复位完成" ("Status")) -> ()  [unwired: 11 in]
              }
              frame 6 {
                n186 = call "浮动通知1.vi"("通知内容"="请按启动扫电机工位主码") -> ()  [unwired: 11 in]
              }
              frame 7 {
                n187 = for {
                  tunnel: w707 -> [w715] mode=indexing
                  n188 = call "Colour -电机.vi"("result"="", "colourRef"=w715) -> ()  [unwired: 9 in, 1 out]
                }
                n189 = global read "Global.vi" "电机结果显示"() -> (w711:refnum<vi>)
                n190 = shared-variable "我的电脑\\Global.lvlib\\工位追溯码"("" ("传感器码")) -> ()  [unwired: 1 in, 1 out]
                n191 = shared-variable "我的电脑\\A17031611.lvlib\\设备状态3"(i16 0 ("设备状态3")) -> ()  [unwired: 1 in, 1 out]
                n192 = property class="Str"(reference=w711, "Value"="..." ("结果显示")) -> (reference out=w710:refnum<vi>)  [unwired: 1 in, 1 out]
                n193 = property class="Str"(reference=w710, "Text.TextColor"=u32 16776960) -> ()  [unwired: 1 in, 2 out]
                n194 = local write "STEP3"("扫管柱码" ("STEP3")) -> ()
              }
              frame 8 {
                n195 = call "浮动通知.vi"("通知内容"="程序停止！" ("Status")) -> ()  [unwired: 11 in]
              }
              frame 9 {
                n196 = call "浮动通知.vi"("通知内容"="套花键中" ("Status")) -> ()  [unwired: 11 in]
              }
              frame 10 {
                n197 = local write "STEP3"("步骤" ("STEP3")) -> ()
                n198 = call "浮动通知.vi"("通知内容"="请安装胶垫弹簧并拍照确认！" ("Status")) -> ()  [unwired: 11 in]
              }
              frame 16 {
                n199 = Index Array(array=w722, index=0 ("索引")) -> (element=w721:refnum<vi>)
                n200 = call "Colour -电机.vi"("result"="等待", "colourRef"=w721) -> ()  [unwired: 9 in, 1 out]
                n201 = call "浮动通知.vi"("通知内容"="请拾取弹簧并安装到位") -> ()  [unwired: 11 in]
              }
              frame 17 {
                n202 = Index Array(array=w729) -> (element #1=w726:refnum<vi>, element #2=w727:refnum<vi>)  [unwired: 2 in]
                n203 = call "Colour -电机.vi"("result"="等待", "colourRef"=w727) -> ()  [unwired: 9 in, 1 out]
                n204 = call "Colour -电机.vi"("result"="OK", "colourRef"=w726) -> ()  [unwired: 9 in, 1 out]
              }
              frame 18 {
                n205 = Index Array(array=w732, index=1 ("索引")) -> (element=w730:refnum<vi>)
                n206 = call "浮动通知.vi"("通知内容"="请拾O型圈") -> ()  [unwired: 11 in]
                n207 = call "Colour -电机.vi"("result"="等待", "colourRef"=w730) -> ()  [unwired: 9 in, 1 out]
              }
              frame 19 {
                n208 = Index Array(array=w739, index #1=1 ("索引")) -> (element #1=w737:refnum<vi>, element #2=w735:refnum<vi>)  [unwired: 1 in]
                n209 = call "Colour -电机.vi"("result"="OK", "colourRef"=w737) -> ()  [unwired: 9 in, 1 out]
                n210 = call "Colour -电机.vi"("result"="等待", "colourRef"=w735) -> ()  [unwired: 9 in, 1 out]
              }
              frame 20 {
                n211 = Index Array(array=w743, index=2 ("索引")) -> (element=w742:refnum<vi>)
                n212 = call "Colour -电机.vi"("result"="等待", "colourRef"=w742) -> ()  [unwired: 9 in, 1 out]
                n213 = call "浮动通知.vi"("通知内容"="请安装胶垫弹簧并拍照确认！" ("Status")) -> ()  [unwired: 11 in]
              }
              frame 30 {
                n214 = Index Array(array=w748, index=2 ("索引")) -> (element=w746:refnum<vi>)
                n215 = call "Colour.vi"("result"="NG", "colourRef"=w746) -> ()  [unwired: 9 in, 1 out]
                n216 = call "浮动通知.vi"("通知内容"="拍照不合格请确认！" ("Status")) -> ()  [unwired: 11 in]
              }
              frame 31 {
                n217 = Index Array(array=w757, index #1=2 ("索引")) -> (element #1=w756:refnum<vi>, element #2=w753:refnum<vi>)  [unwired: 1 in]
                n218 = call "Colour -电机.vi"("result"="OK", "colourRef"=w756) -> ()  [unwired: 9 in, 1 out]
                n219 = call "Colour -电机.vi"("result"="等待", "colourRef"=w753) -> ()  [unwired: 9 in, 1 out]
                n220 = local write "STEP3"("扫电机码" ("STEP3")) -> ()
                n221 = global read "Global.vi" "产品型号"() -> (w751:string)
                n222 = case shown="默认" w751 {
                  frame Default {
                    n223 = local read "电机步骤"() -> (w759:T3)
                    n224 = Increment(x=w759) -> (x+1=w760:T3)
                    n225 = local write "电机步骤"(w760) -> ()
                  }
                  frame "R567X" {
                    n226 = local write "电机步骤"(T3."预拧紧1" ("电机步骤")) -> ()
                  }
                }
              }
              frame 35 {
                n227 = case shown="2" w762 {
                  tunnel: w764 -> [_ w769]
                  frame 0, Default {
                  }
                  frame 2 {
                    n228 = Index Array(array=w769, index #1=0 ("索引")) -> (element #1=w768:refnum<vi>, element #2=w766:refnum<vi>)  [unwired: 1 in]
                    n229 = call "Colour -电机.vi"("result"="OK", "colourRef"=w768) -> ()  [unwired: 9 in, 1 out]
                    n230 = call "Colour -电机.vi"("result"="等待", "colourRef"=w766) -> ()  [unwired: 9 in, 1 out]
                  }
                }
                n231 = call "浮动通知.vi"("通知内容"="请安装固定螺栓1并确认扭矩！" ("Status")) -> ()  [unwired: 11 in]
              }
              frame 36 {
                n232 = case shown="2" w772 {
                  tunnel: w771 -> [w774 w787 w791]
                  frame 1 {
                    n233 = Index Array(array=w774, index=1 ("索引")) -> (element=w781:refnum<vi>)
                    n234 = Index Array(array=w774, index=4 ("索引")) -> (element=w775:refnum<vi>)
                    n235 = call "Colour.vi"("result"="OK", "colourRef"=w781) -> ()  [unwired: 9 in, 1 out]
                    n236 = call "Colour.vi"("result"="等待", "colourRef"=w775) -> ()  [unwired: 9 in, 1 out]
                    n237 = call "浮动通知.vi"("通知内容"="请按启动拍照确认电机方向！" ("Status")) -> ()  [unwired: 11 in]
                    n238 = shared-variable "我的电脑\\A17031611.lvlib\\设备状态1"(i16 70 ("设备状态")) -> ()  [unwired: 1 in, 1 out]
                  }
                  frame 2 {
                    n239 = Index Array(array=w787, index #1=0 ("索引")) -> (element #1=w785:refnum<vi>, element #2=w783:refnum<vi>)  [unwired: 2 in, 1 out]
                    n240 = call "Colour -电机.vi"("result"="OK", "colourRef"=w785) -> ()  [unwired: 9 in, 1 out]
                    n241 = call "Colour -电机.vi"("result"="等待", "colourRef"=w783) -> ()  [unwired: 9 in, 1 out]
                    n242 = call "浮动通知.vi"("通知内容"="请安装固定螺栓1并确认扭矩！" ("Status")) -> ()  [unwired: 11 in]
                  }
                  frame Default {
                    n243 = Index Array(array=w791, index #1=1 ("索引")) -> (element #1=w795:refnum<vi>, element #2=w796:refnum<vi>)  [unwired: 1 in]
                    n244 = call "Colour.vi"("result"="OK", "colourRef"=w795) -> ()  [unwired: 9 in, 1 out]
                    n245 = call "浮动通知.vi"("通知内容"="请安装固定螺栓2并确认扭矩！" ("Status")) -> ()  [unwired: 11 in]
                    n246 = call "Colour.vi"("result"="等待", "colourRef"=w796) -> ()  [unwired: 9 in, 1 out]
                    n247 = shared-variable "我的电脑\\A17031611.lvlib\\设备状态3"(i16 40 ("设备状态")) -> ()  [unwired: 1 in, 1 out]
                  }
                }
              }
              frame 40 {
                n248 = Index Array(array=w799, index=3 ("索引")) -> (element=w797:refnum<vi>)
                n249 = call "Colour -电机.vi"("result"="等待", "colourRef"=w797) -> ()  [unwired: 9 in, 1 out]
                n250 = call "浮动通知.vi"("通知内容"="请预拧紧电机螺栓1！" ("Status")) -> ()  [unwired: 11 in]
              }
              frame 41 {
                n251 = Index Array(array=w807, index #1=3 ("索引")) -> (element #1=w805:refnum<vi>, element #2=w803:refnum<vi>)  [unwired: 1 in]
                n252 = call "Colour -电机.vi"("result"="OK", "colourRef"=w805) -> ()  [unwired: 9 in, 1 out]
                n253 = call "Colour -电机.vi"("result"="等待", "colourRef"=w803) -> ()  [unwired: 9 in, 1 out]
                n254 = shared-variable "我的电脑\\A17031611.lvlib\\设备状态3"(i16 42 ("设备状态3")) -> ()  [unwired: 1 in, 1 out]
              }
              frame 42 {
                n255 = Index Array(array=w811, index=4 ("索引")) -> (element=w810:refnum<vi>)
                n256 = call "浮动通知.vi"("通知内容"="请预拧紧电机螺栓2！" ("Status")) -> ()  [unwired: 11 in]
                n257 = call "Colour -电机.vi"("result"="等待", "colourRef"=w810) -> ()  [unwired: 9 in, 1 out]
              }
              frame 43 {
                n258 = Index Array(array=w819, index #1=4 ("索引")) -> (element #1=w817:refnum<vi>, element #2=w815:refnum<vi>)  [unwired: 1 in]
                n259 = call "Colour -电机.vi"("result"="等待", "colourRef"=w815) -> ()  [unwired: 9 in, 1 out]
                n260 = call "Colour -电机.vi"("result"="OK", "colourRef"=w817) -> ()  [unwired: 9 in, 1 out]
                n261 = shared-variable "我的电脑\\A17031611.lvlib\\设备状态3"(i16 44 ("设备状态3")) -> ()  [unwired: 1 in, 1 out]
              }
              frame 44 {
                n262 = Index Array(array=w823, index=5 ("索引")) -> (element=w822:refnum<vi>)
                n263 = call "浮动通知.vi"("通知内容"="请确认电机螺栓1扭矩！" ("Status")) -> ()  [unwired: 11 in]
                n264 = call "Colour -电机.vi"("result"="等待", "colourRef"=w822) -> ()  [unwired: 9 in, 1 out]
              }
              frame 45 {
                n265 = Index Array(array=w831, index #1=5 ("索引")) -> (element #1=w830:refnum<vi>, element #2=w827:refnum<vi>)  [unwired: 1 in]
                n266 = shared-variable "我的电脑\\A17031611.lvlib\\设备状态3"(i16 46 ("设备状态3")) -> ()  [unwired: 1 in, 1 out]
                n267 = call "Colour -电机.vi"("result"="等待", "colourRef"=w827) -> ()  [unwired: 9 in, 1 out]
                n268 = call "Colour -电机.vi"("result"="OK", "colourRef"=w830) -> ()  [unwired: 9 in, 1 out]
              }
              frame 46 {
                n269 = Index Array(array=w836, index=6 ("索引")) -> (element=w835:refnum<vi>)
                n270 = call "Colour -电机.vi"("result"="等待", "colourRef"=w835) -> ()  [unwired: 9 in, 1 out]
                n271 = call "浮动通知.vi"("通知内容"="请确认电机螺栓2扭矩！" ("Status")) -> ()  [unwired: 11 in]
              }
              frame 47 {
                n272 = Index Array(array=w843, index #1=6 ("索引")) -> (element #1=w842:refnum<vi>, element #2=w839:refnum<vi>)  [unwired: 1 in]
                n273 = shared-variable "我的电脑\\A17031611.lvlib\\设备状态3"(i16 70 ("设备状态3")) -> ()  [unwired: 1 in, 1 out]
                n274 = call "Colour -电机.vi"("result"="等待", "colourRef"=w839) -> ()  [unwired: 9 in, 1 out]
                n275 = call "Colour -电机.vi"("result"="OK", "colourRef"=w842) -> ()  [unwired: 9 in, 1 out]
              }
              frame 51 {
                n276 = case shown="2" w846 {
                  tunnel: w845 -> [_ _ w851]
                  frame 0, 1 {
                  }
                  frame 2 {
                    n277 = call "浮动通知.vi"("通知内容"="请按启动按钮拍照确认！" ("Status")) -> ()  [unwired: 11 in]
                    n278 = shared-variable "我的电脑\\A17031611.lvlib\\设备状态3"(i16 70 ("设备状态")) -> ()  [unwired: 1 in, 1 out]
                  }
                  frame Default {
                    n279 = Index Array(array=w851, index #1=2 ("索引")) -> (element #1=w855:refnum<vi>, element #2=w852:refnum<vi>)  [unwired: 1 in]
                    n280 = call "浮动通知.vi"("通知内容"="请按启动按钮拍照确认！" ("Status")) -> ()  [unwired: 11 in]
                    n281 = call "Colour.vi"("result"="OK", "colourRef"=w855) -> ()  [unwired: 9 in, 1 out]
                    n282 = call "Colour.vi"("result"="等待", "colourRef"=w852) -> ()  [unwired: 9 in, 1 out]
                    n283 = shared-variable "我的电脑\\A17031611.lvlib\\设备状态3"(i16 70 ("设备状态")) -> ()  [unwired: 1 in, 1 out]
                  }
                }
              }
              frame 61 {
                n284 = case shown="默认" w858 {
                  tunnel: w857 -> [w863 _]
                  frame Default {
                    n285 = Index Array(array=w863, index #1=3 ("索引")) -> (element #1=w865:refnum<vi>, element #2=w866:refnum<vi>)  [unwired: 1 in]
                    n286 = call "Colour.vi"("result"="OK", "colourRef"=w865) -> ()  [unwired: 9 in, 1 out]
                    n287 = call "Colour.vi"("result"="等待", "colourRef"=w866) -> ()  [unwired: 9 in, 1 out]
                    n288 = call "浮动通知.vi"("通知内容"="请按启动拍照确认！" ("Status")) -> ()  [unwired: 11 in]
                    n289 = shared-variable "我的电脑\\A17031611.lvlib\\设备状态3"(i16 70 ("设备状态")) -> ()  [unwired: 1 in, 1 out]
                  }
                  frame 0..2 {
                  }
                }
              }
              frame 70 {
                n290 = Index Array(array=w869, index=7 ("索引")) -> (element=w868:refnum<vi>)
                n291 = call "浮动通知.vi"("通知内容"="请按启动拍照确认！" ("Status")) -> ()  [unwired: 11 in]
                n292 = call "Colour -电机.vi"("result"="等待", "colourRef"=w868) -> ()  [unwired: 9 in, 1 out]
              }
              frame 80 {
                n293 = Index Array(array=w875, index=7 ("索引")) -> (element=w874:refnum<vi>)
                n294 = call "浮动通知.vi"("通知内容"="电机拍照不合格请检查！") -> ()  [unwired: 11 in]
                n295 = call "Colour -电机.vi"("result"="NG", "colourRef"=w874) -> ()  [unwired: 9 in, 1 out]
              }
              frame 81 {
                n296 = Index Array(array=w882, index #1=7 ("索引")) -> (element #1=w880:refnum<vi>, element #2=w878:refnum<vi>)  [unwired: 1 in]
                n297 = shared-variable "我的电脑\\A17031611.lvlib\\设备状态3"(i16 90 ("设备状态3")) -> ()  [unwired: 1 in, 1 out]
                n298 = call "Colour -电机.vi"("result"="OK", "colourRef"=w880) -> ()  [unwired: 9 in, 1 out]
                n299 = call "Colour -电机.vi"("result"="等待", "colourRef"=w878) -> ()  [unwired: 9 in, 1 out]
              }
              frame 90 {
                n300 = Index Array(array=w886, index=8 ("索引")) -> (element=w884:refnum<vi>)
                n301 = call "浮动通知.vi"("通知内容"="请给固定螺栓涂色标！" ("Status")) -> ()  [unwired: 11 in]
                n302 = call "Colour -电机.vi"("result"="等待", "colourRef"=w884) -> ()  [unwired: 9 in, 1 out]
              }
              frame 91 {
                n303 = Index Array(array=w894, index #1=8 ("索引")) -> (element #1=w893:refnum<vi>, element #2=w890:refnum<vi>)  [unwired: 1 in]
                n304 = shared-variable "我的电脑\\A17031611.lvlib\\设备状态3"(i16 100 ("设备状态3")) -> ()  [unwired: 1 in, 1 out]
                n305 = call "Colour -电机.vi"("result"="OK", "colourRef"=w893) -> ()  [unwired: 9 in, 1 out]
                n306 = call "Colour -电机.vi"("result"="等待", "colourRef"=w890) -> ()  [unwired: 9 in, 1 out]
              }
              frame 100 {
                n307 = Index Array(array=w898, index=9 ("索引")) -> (element=w896:refnum<vi>)
                n308 = call "Colour -电机.vi"("result"="等待", "colourRef"=w896) -> ()  [unwired: 9 in, 1 out]
                n309 = call "浮动通知.vi"("通知内容"="请安装轧带并取走工件" ("Status")) -> ()  [unwired: 11 in]
              }
              frame 101 {
                n310 = Index Array(array=w904, index=9 ("索引")) -> (element=w902:refnum<vi>)
                n311 = call "Colour -电机.vi"("result"="OK", "colourRef"=w902) -> ()  [unwired: 9 in, 1 out]
                n312 = shared-variable "我的电脑\\A17031611.lvlib\\设备状态3"(i16 110 ("设备状态3")) -> ()  [unwired: 1 in, 1 out]
              }
              frame 200 {
                n313 = global read "Global1.vi" "联机模式"() -> (w906:enum16{"单机", "联网"})
                n314 = Wait (ms)(milliseconds to wait=u32 100 ("等待时间（毫秒）")) -> ()  [unwired: 1 out]
                n315 = case shown="\"联网\"" w906 {
                  frame "单机", Default {
                    n316 = global read "Global.vi" "检测结果"() -> (w915:refnum<vi>)
                    n317 = call "浮动通知.vi"("通知内容"="产品合格！" ("Status")) -> ()  [unwired: 11 in]
                    n318 = call "Colour.vi"("result"="OK", "colourRef"=w915) -> ()  [unwired: 9 in, 1 out]
                    n319 = global read "Global.vi" "电机结果显示"() -> (w912:refnum<vi>)
                    n320 = local write "STEP3"("初始化" ("STEP3")) -> ()
                    n321 = property class="Str"(reference=w912, "Value"="OK" ("结果显示")) -> (reference out=w911:refnum<vi>)  [unwired: 1 in, 1 out]
                    n322 = property class="Str"(reference=w911, "Text.TextColor"=u32 6618880) -> ()  [unwired: 1 in, 2 out]
                  }
                  frame "联网" {
                    n323 = global read "Global.vi" "检测结果"() -> (w918:refnum<vi>)
                    n324 = global write "Global1.vi" "电机工位生产结果"("OK" ("电机工位生产结果")) -> ()
                    n325 = call "浮动通知.vi"("通知内容"="产品合格！" ("Status")) -> ()  [unwired: 11 in]
                    n326 = call "Colour -电机.vi"("result"="OK", "colourRef"=w918) -> ()  [unwired: 9 in, 1 out]
                    n327 = global read "Global.vi" "电机结果显示"() -> (w924:refnum<vi>)
                    n328 = local write "STEP3"("录入数据库" ("STEP3")) -> ()
                    n329 = property class="Str"(reference=w924, "Value"="OK" ("结果显示")) -> (reference out=w921:refnum<vi>)  [unwired: 1 in, 1 out]
                    n330 = property class="Str"(reference=w921, "Text.TextColor"=u32 6618880) -> ()  [unwired: 1 in, 2 out]
                  }
                }
              }
              frame 201 {
                n331 = global read "Global.vi" "检测结果"() -> (w930:refnum<vi>)
                n332 = call "Colour.vi"("result"="NG", "colourRef"=w930) -> ()  [unwired: 9 in, 1 out]
                n333 = call "浮动通知.vi"("通知内容"="产品不合格！" ("Status")) -> ()  [unwired: 11 in]
                n334 = global read "Global.vi" "电机结果显示"() -> (w929:refnum<vi>)
                n335 = property class="Str"(reference=w929, "Value"="NG" ("结果显示")) -> (reference out=w928:refnum<vi>)  [unwired: 1 in, 1 out]
                n336 = property class="Str"(reference=w928, "Text.TextColor"=u32 16711680) -> ()  [unwired: 1 in, 2 out]
              }
              frame 999 {
                n337 = Index Array(array=w934, index #1=0 ("索引")) -> (element #1=w942:refnum<vi>, element #2=w943:refnum<vi>, element #3=w935:refnum<vi>, element #4=w932:refnum<vi>)  [unwired: 3 in]
                n338 = call "Colour.vi"("result"="", "colourRef"=w935) -> ()  [unwired: 9 in, 1 out]
                n339 = call "Colour.vi"("result"="", "colourRef"=w932) -> ()  [unwired: 9 in, 1 out]
                n340 = call "Colour.vi"("result"="NG", "colourRef"=w943) -> ()  [unwired: 9 in, 1 out]
                n341 = call "Colour.vi"("result"="OK", "colourRef"=w942) -> ()  [unwired: 9 in, 1 out]
                n342 = call "浮动通知.vi"("通知内容"="请重新安装固定螺栓！" ("Status")) -> ()  [unwired: 11 in]
                n343 = shared-variable "我的电脑\\A17031611.lvlib\\设备状态3"(i16 40 ("设备状态")) -> ()  [unwired: 1 in, 1 out]
              }
              frame 1024 {
                n344 = call "浮动通知.vi"("通知内容"="急停！" ("Status")) -> ()  [unwired: 11 in]
                n345 = global read "Global.vi" "电机程序自动"() -> (w945:refnum<vi>)
                n346 = property class="Bool"(reference=w945, "Value"=FALSE) -> ()  [unwired: 1 in, 2 out]
              }
              frame 3721 {
                n347 = local write "STEP3"("不合格锁定" ("STEP")) -> ()
                n348 = call "浮动通知.vi"("通知内容"="产品不合格程序锁定！" ("Status")) -> ()  [unwired: 11 in]
              }
              frame 3722 {
                n349 = global read "Global.vi" "电机程序自动"() -> (w950:refnum<vi>)
                n350 = call "浮动通知.vi"("通知内容"="授权成功，请复位！" ("Status")) -> ()  [unwired: 11 in]
                n351 = property class="Bool"(reference=w950, "Value"=FALSE) -> ()  [unwired: 1 in, 2 out]
              }
              frame 3723 {
                n352 = call "浮动通知.vi"("通知内容"="请取出不合格产品并摆放至不合格品区！" ("Status")) -> ()  [unwired: 11 in]
              }
              frame Default {
              }
            }
          }
          frame "录入数据库" {
            n353 = stacked-sequence {
              frame #0 {
                n354 = Get Date/Time String(date format (0)=enum16{"short", "long", "abbreviated"}."short" ("日期格式(0)"), want seconds? (F)=FALSE ("需要秒？(F)")) -> (date string=w962:string, time string=w963:string)  [unwired: 1 in]
                n355 = global read "Global1.vi" "电机工位生产结果"() -> (w957:string)
                n356 = global read "Global1.vi" "DEVICE_ID"() -> (w966:string)
                n357 = global read "Global1.vi" "USER_ID"() -> (w964:string)
                n358 = global read "Global1.vi" "CODE_ID"() -> (w965:string)
                n359 = Concatenate Strings(w962, " " ("字符串"), w963) -> (w958:string)
                n360 = Decimal String To Number(string=w966, default (0L)=i64 0 ("默认(0 I32)")) -> (number=w955:i64)  [unwired: 1 in, 1 out]
                n361 = Decimal String To Number(string=w964, default (0L)=i64 0 ("默认(0 I32)")) -> (number=w954:i64)  [unwired: 1 in, 1 out]
                n362 = Decimal String To Number(string=w965, default (0L)=i64 0 ("默认(0 I32)")) -> (number=w953:i64)  [unwired: 1 in, 1 out]
                n363 = global read "Global1.vi" "联机模式"() -> (w973:enum16{"单机", "联网"})
                n364 = Search and Replace String(replace all?=TRUE ("替换全部？(F)"), input string=w958, search string="/" ("替换字符串(\"\")"), replace string="-" ("替换字符串(\"\")")) -> (result string=w956:string)  [unwired: 4 in, 3 out]
                n365 = Bundle(w955, w954, w953, "电机工位生产结果"=w957, "result string"=w956) -> (w979:T4)  [unwired: 1 in]
                n366 = call "GetSQLstring.vi"("联机模式"=w973) -> ("错误输出"=w976:errorcluster, "连接字符串"=w975:string)  [unwired: 9 in]
                n367 = Build Array(w979) -> (w980:T5)
                n368 = call-poly <vilib>:"DB Tools Open Connection.vi"("error in (no error)"=w976, "connection information"=w975) -> ("error out"=w974:errorcluster, "connection reference"=w977:T6)  [unwired: 6 in]
                n369 = for {
                  tunnel: w980 -> [w985] mode=indexing
                  tunnel: w977 -> [w983]
                  shift-right: [w981] -> w978
                  shift-left: w974 -> [w988]
                  w984 = string[] ["DEVICE_ID", "USER_ID", "CODE_ID", "RESULT_VALUE", "RESULT_TIME"] ("columns")
                  w986 = "Result" ("table")
                  n370 = call <vilib>:"DB Tools Insert Data.vi"("data"=w985, "error in (no error)"=w988, "columns"=w984, "table"=w986, "connection reference"=w983) -> ("error out"=w987:errorcluster, "connection reference out"=w982:T6)  [unwired: 5 in]
                  n371 = case shown="错误" w987 {
                    selector: w987 -> [w989 w1010]
                    tunnel: w984 -> [_ w1007]
                    tunnel: w982 -> [w990 w999]
                    tunnel: w986 -> [_ w1011]
                    tunnel: w985 -> [_ w1003]
                    tunnel: [w990 w998] -> _
                    tunnel: [w989 w997] -> w981
                    frame No Error {
                    }
                    frame Error {
                      n372 = Array Subset(array=w1007, index=3 ("长度"), length=2 ("长度")) -> (w1008:string[])
                      n373 = Unbundle(w1003) -> (w992:i64, w995:i64, "电机工位生产结果"=w1002:string, "result string"=w1001:string)  [unwired: 1 out]
                      n374 = Number To Decimal String(number=w995) -> (decimal integer string=w996:string)  [unwired: 1 in]
                      n375 = Number To Decimal String(number=w992) -> (decimal integer string=w991:string)  [unwired: 1 in]
                      n376 = Concatenate Strings("WHERE CODE_ID =" ("condition"), w996, "AND DEVICE_ID = ", w991) -> (w1004:string)
                      n377 = Bundle("电机工位生产结果"=w1002, "result string"=w1001) -> (w1000:T7)  [unwired: 1 in]
                      n378 = call <vilib>:"Clear Errors.vi"("error in (no error)"=w1010) -> ("error out"=w1009:errorcluster)  [unwired: 5 in, 1 out]
                      n379 = call <vilib>:"DB Tools Update Data.vi"("condition"=w1004, "data"=w1000, "error in (no error)"=w1009, "columns"=w1008, "table"=w1011, "connection reference"=w999) -> ("error out"=w997:errorcluster, "connection reference out"=w998:T6)  [unwired: 4 in]
                    }
                  }
                }
                n380 = call <vilib>:"Simple Error Handler.vi"("error in (no error)"=w978) -> ()  [unwired: 4 in, 5 out]
              }
              frame #1 {
                n381 = global read "Global1.vi" "电机码"() -> (w1012:string)
                n382 = global read "Global1.vi" "CODE_ID"() -> (w1013:string)
                n383 = Format Into String(format string="UPDATE\ndbo.[Code]\nSET dbo.[Code].CODE_MOTOR = '%s'\n\nWHERE\ndbo.[Code].CODE_ID = %s\n" ("格式字符串"), w1012, w1013) -> (resulting string=w1016:string)  [unwired: 2 in, 1 out]
                n384 = call "SQL_query.vi"("SQL query"=w1016, "联机模式"=enum16{"单机", "联网"}."联网") -> ()  [unwired: 1 in, 3 out]
              }
              frame #2 {
                n385 = local write "STEP3"("初始化" ("STEP")) -> ()
                n386 = call "浮动通知.vi"("通知内容"="电机工位数据录入成功！" ("Status")) -> ()  [unwired: 11 in]
                n387 = Wait (ms)(milliseconds to wait=u32 500 ("等待时间（毫秒）")) -> ()  [unwired: 1 out]
              }
            }
          }
          frame "不合格锁定" {
            n388 = call "临时授权.vi"() -> ("授权成功"=w1021:bool)  [unwired: 11 in]
            n389 = case shown="真" w1021 {
              frame False {
              }
              frame True {
                n390 = local write "STEP3"("报表" ("STEP")) -> ()
                n391 = shared-variable "我的电脑\\A17031611.lvlib\\设备状态1"(i16 3722 ("设备状态")) -> ()  [unwired: 1 in, 1 out]
              }
            }
            n392 = Wait (ms)(milliseconds to wait=u32 100 ("等待时间（毫秒）")) -> ()  [unwired: 1 out]
          }
          frame "报表" {
            n393 = call "浮动通知.vi"("通知内容"="报表生成中" ("Status")) -> ()  [unwired: 11 in]
            n394 = shared-variable "我的电脑\\Global.lvlib\\工位追溯码"() -> (w1033:string)  [unwired: 1 in, 1 out]
            n395 = Index Array(array="判定结果", index (col)=1 ("禁用的索引 (列)")) -> (element=w1028:bool[])  [unwired: 1 in]
            n396 = And Array Elements(Boolean array=w1028) -> (logical AND=w1025:bool)
            n397 = shared-variable "我的电脑\\Global.lvlib\\联机模式"() -> (w1030:i16)  [unwired: 1 in, 1 out]
            n398 = call "Report_A170316-11.vi"("文件重命名"=TRUE, "文件名称"=w1033, "布尔数组"="判定结果") -> ("error out"=w1031:errorcluster)  [unwired: 8 in]
            n399 = case shown="真" w1025 {
              frame False {
              }
              frame True {
                n400 = global read "Global.vi" "电机生产数量"() -> (w1042:refnum<vi>)
                n401 = property class="Num"(reference=w1042) -> (reference out=w1041:refnum<vi>, error out=w1040:errorcluster, "Value"=w1039:variant)  [unwired: 1 in]
                n402 = Variant To Data(type=u32 0, Variant=w1039) -> (data=w1038:u32)  [unwired: 1 in, 1 out]
                n403 = Increment(x=w1038) -> (x+1=w1037:u32)
                n404 = property class="Num"(reference=w1041, error in=w1040, "Value"=w1037) -> ()  [unwired: 2 out]
              }
            }
            n405 = case shown="0, 默认" w1030 {
              tunnel: w1031 -> [_ w1043]
              frame 0, Default {
              }
              frame 1 {
                n406 = call "上传数据库.vi"("错误输入"=w1043) -> ()  [unwired: 10 in, 1 out]
              }
            }
            n407 = shared-variable "我的电脑\\A17031611.lvlib\\设备状态1"() -> (w1024:i16)  [unwired: 1 in, 1 out]
            n408 = case shown="3721..3723" w1024 {
              frame Default {
                n409 = local write "STEP3"("初始化" ("STEP")) -> ()
              }
              frame 3721..3723 {
                n410 = local write "STEP3"("等待" ("STEP")) -> ()
              }
            }
          }
          frame "步骤" {
            n411 = case shown="\"安装弹簧\", 默认" "电机步骤" {
              selector: "电机步骤" -> [w1047 _]
              tunnel: [w1046 "等待"] -> w1044
              frame "安装弹簧", Default {
                n412 = global read "Global.vi" "电机安装"() -> (w1049:bool[])
                n413 = Index Array(array=w1049, index=w1047) -> (element=w1048:bool)
                n414 = case shown="真" w1048 {
                  tunnel: w1047 -> [_ w1054]
                  tunnel: ["步骤" w1053] -> w1046
                  frame False {
                    n415 = local read "电机步骤"() -> (w1052:T3)
                    n416 = Increment(x=w1052) -> (x+1=w1051:T3)
                    n417 = local write "电机步骤"(w1051) -> ()
                  }
                  frame True {
                    n418 = case shown="\"预拧紧1\"" w1054 {
                      tunnel: ["自动" "自动" "自动" "自动" "自动" "自动" "自动" "等待" "等待" "等待"] -> w1053
                      frame "安装弹簧", Default {
                        n419 = shared-variable "我的电脑\\A17031611.lvlib\\设备状态3"(i16 16 ("设备状态")) -> ()  [unwired: 1 in, 1 out]
                      }
                      frame "安装O型圈" {
                        n420 = shared-variable "我的电脑\\A17031611.lvlib\\设备状态3"(i16 18 ("设备状态")) -> ()  [unwired: 1 in, 1 out]
                      }
                      frame "安装弹性垫圈" {
                        n421 = shared-variable "我的电脑\\A17031611.lvlib\\设备状态3"(i16 20 ("设备状态")) -> ()  [unwired: 1 in, 1 out]
                      }
                      frame "预拧紧1" {
                        n422 = shared-variable "我的电脑\\A17031611.lvlib\\设备状态3"(i16 40 ("设备状态3")) -> ()  [unwired: 1 in, 1 out]
                      }
                      frame "预拧紧2" {
                        n423 = shared-variable "我的电脑\\A17031611.lvlib\\设备状态3"(i16 42 ("设备状态控制字")) -> ()  [unwired: 1 in, 1 out]
                      }
                      frame "电机1" {
                        n424 = shared-variable "我的电脑\\A17031611.lvlib\\设备状态3"(i16 40 ("设备状态控制字")) -> ()  [unwired: 1 in, 1 out]
                      }
                      frame "电机2" {
                        n425 = shared-variable "我的电脑\\A17031611.lvlib\\设备状态3"(i16 42 ("设备状态控制字")) -> ()  [unwired: 1 in, 1 out]
                      }
                      frame "电机拍照" {
                        n426 = shared-variable "我的电脑\\A17031611.lvlib\\设备状态3"(i16 70 ("设备状态控制字")) -> ()  [unwired: 1 in, 1 out]
                      }
                      frame "涂色标" {
                        n427 = shared-variable "我的电脑\\A17031611.lvlib\\设备状态3"(i16 90 ("设备状态控制字")) -> ()  [unwired: 1 in, 1 out]
                      }
                      frame "安装轧带取走工件" {
                        n428 = shared-variable "我的电脑\\A17031611.lvlib\\设备状态3"(i16 100 ("设备状态控制字")) -> ()  [unwired: 1 in, 1 out]
                      }
                    }
                  }
                }
              }
              frame "完成" {
                n429 = shared-variable "我的电脑\\A17031611.lvlib\\设备状态3"(i16 200 ("设备状态控制字")) -> ()  [unwired: 1 in, 1 out]
              }
            }
            n430 = local write "STEP3"(w1044) -> ()
          }
        }
        n431 = global read "Global.vi" "程序关闭"() -> (w550:bool)
      }
      n432 = while {
        stop <- w48 stop-if-true
        n433 = Wait Until Next ms Multiple(millisecond multiple=u32 50 ("等待时间（毫秒）")) -> ()  [unwired: 1 out]
        n434 = case shown="\"步骤\"" "STEP2" {
          frame "等待", Default {
            n435 = local write "STEP2"("自动" ("STEP")) -> ()
            n436 = Wait (ms)(milliseconds to wait=u32 200 ("等待时间（毫秒）")) -> ()  [unwired: 1 out]
          }
          frame "手动" {
            n437 = global read "Global.vi" "ECU自动"() -> (w177:refnum<vi>)
            n438 = shared-variable "我的电脑\\A17031611.lvlib\\设备状态1"(u16 0 ("设备状态")) -> ()  [unwired: 1 in, 1 out]
            n439 = shared-variable "我的电脑\\A17031611.lvlib\\设备状态2"(u16 0 ("设备状态")) -> ()  [unwired: 1 in, 1 out]
            n440 = property class="Bool (严格)"(reference=w177, "Value"=FALSE) -> ()  [unwired: 1 in, 2 out]
            n441 = local write "STEP2"("等待" ("STEP")) -> ()
            n442 = local write "STEP1"("等待" ("STEP1")) -> ()
            n443 = Wait (ms)(milliseconds to wait=u32 100 ("等待时间（毫秒）")) -> ()  [unwired: 1 out]
            n444 = global read "Global.vi" "电机程序自动"() -> (w176:refnum<vi>)
            n445 = shared-variable "我的电脑\\A17031611.lvlib\\设备状态3"(u16 0 ("设备状态")) -> ()  [unwired: 1 in, 1 out]
            n446 = property class="Bool"(reference=w176, "Value"=FALSE) -> ()  [unwired: 1 in, 2 out]
          }
          frame "初始化" {
            n447 = stacked-sequence {
              frame #0 {
                w187 = enum16{"录入", "清空"}."清空" ("功能")
                n448 = global read "Global.vi" "安装支架生产数量"() -> (w179:refnum<vi>)
                n449 = shared-variable "我的电脑\\Global.lvlib\\工位追溯码"("" ("传感器码")) -> ()  [unwired: 1 in, 1 out]
                n450 = call "物料信息录入.vi"("功能"=w187) -> ("错误输出"=w186:errorcluster)  [unwired: 14 in]
                n451 = call "质量信息录入.vi"("功能"=w187, "错误输入（无错误）"=w186) -> ("错误输出"=w188:errorcluster)  [unwired: 13 in]
                n452 = property class="Num"(reference=w179, "Value"=0 ("磨合次数")) -> ()  [unwired: 1 in, 2 out]
                n453 = call "不合格信息录入.vi"("功能"=w187, "错误输入（无错误）"=w188) -> ()  [unwired: 13 in, 1 out]
                n454 = global read "Global.vi" "ECU自动"() -> (w184:refnum<vi>)
                n455 = global read "Global.vi" "检测结果"() -> (w182:refnum<vi>)
                n456 = property class="Bool (严格)"(reference=w184, "Value"=TRUE) -> ()  [unwired: 1 in, 2 out]
                n457 = shared-variable "我的电脑\\A17031611.lvlib\\设备状态2"(i16 6 ("设备状态")) -> ()  [unwired: 1 in, 1 out]
                n458 = call "Colour.vi"("result"="", "colourRef"=w182) -> ()  [unwired: 9 in, 1 out]
              }
              frame #1 {
                n459 = local write "ECU步骤"(T2."控制器安装螺栓1" ("ECU步骤")) -> ()
              }
              frame #2 {
                n460 = local write "STEP2"("等待" ("STEP2")) -> ()
              }
            }
          }
          frame "扫主码" {
            n461 = stacked-sequence {
              frame #0 {
                w192 = "请扫ECU工位主码！" ("提示信息")
                n462 = call "浮动通知2.vi"("通知内容"=w192) -> ()  [unwired: 11 in]
                n463 = call "输入框.vi"("提示信息"=w192) -> ("条形码输出"=w193:string)
                n464 = case shown="\"\", 默认" w193 {
                  selector: w193 -> [w194 _]
                  tunnel: [w195 "手动"] -> w191
                  frame "", Default {
                    n465 = shared-variable "我的电脑\\Global.lvlib\\工位追溯码_ECU"(w194) -> ()  [unwired: 1 in, 1 out]
                    n466 = global write "Global1.vi" "工位追溯码_ECU"(w194) -> ()
                    n467 = global read "Global1.vi" "联机模式"() -> (w196:enum16{"单机", "联网"})
                    n468 = case shown="\"单机\", 默认" w196 {
                      tunnel: w194 -> [_ w200]
                      tunnel: ["控制器扫码" ("State(s) in Front (\"\")") w199] -> w195
                      frame "单机", Default {
                        n469 = Wait (ms)(milliseconds to wait=u32 100 ("等待时间（毫秒）")) -> ()  [unwired: 1 out]
                      }
                      frame "联网" {
                        n470 = stacked-sequence {
                          tunnel: w200 -> [w201 _ _]
                          tunnel: [_ _ w221] -> w199
                          frame #0 {
                            n471 = global read "Global1.vi" "PRODUCT_ID_ECU"() -> (w205:string)
                            n472 = Format Into String "格式化写入字符串"(format string="SELECT\ndbo.[Code].CODE_ID\nFROM\ndbo.[Code]\nWHERE\ndbo.[Code].CODE_MAIN = '%s'\nAND\ndbo.[Code].PRODUCT_ID = %s\n" ("格式字符串"), w201, w205) -> (resulting string=w207:string)  [unwired: 2 in, 1 out]
                            n473 = call "SQL_query.vi"("SQL query"=w207, "联机模式"=enum16{"单机", "联网"}."联网") -> ("data"=w210:string[][])  [unwired: 1 in, 2 out]
                            n474 = Index Array(array=w210, index (row)=0 ("索引 (行)")) -> (element=w209:string[])  [unwired: 1 in]
                            n475 = Index Array(array=w209, index=0 ("索引")) -> (element=w202:string)
                            n476 = global write "Global1.vi" "CODE_ID_ECU"(w202) -> ()
                          }
                          frame #1 {
                            n477 = global read "Global1.vi" "前序DEVICE_ID_ECU"() -> (w211:string)
                            n478 = global read "Global1.vi" "CODE_ID_ECU"() -> (w212:string)
                            n479 = Format Into String(format string="SELECT\ndbo.[Result].RESULT_VALUE\nFROM\ndbo.[Result]\nWHERE\ndbo.[Result].DEVICE_ID = %s\nAND\ndbo.[Result].CODE_ID = %s\n" ("格式字符串"), w211, w212) -> (resulting string=w214:string)  [unwired: 2 in, 1 out]
                            n480 = call "SQL_query.vi"("SQL query"=w214, "联机模式"=enum16{"单机", "联网"}."联网") -> ("data"=w220:string[][])  [unwired: 1 in, 2 out]
                            n481 = Index Array(array=w220, index (row)=0 ("索引 (行)")) -> (element=w219:string[])  [unwired: 1 in]
                            n482 = Index Array(array=w219, index=0 ("索引")) -> (element=w213:string)
                            n483 = local write "前序OK？_ECU"(w213) -> ()
                          }
                          frame #2 {
                            n484 = local read "前序OK？_ECU"() -> (w222:string)
                            n485 = case shown="\"OK\"" w222 {
                              tunnel: ["控制器扫码" "自动" "自动"] -> w221
                              frame "OK" {
                                n486 = global read "Global.vi" "ECU前序显示字"() -> (w226:refnum<vi>)
                                n487 = global read "Global1.vi" "ECU上序状态"() -> (w225:refnum<vi>)
                                n488 = property class="Str"(reference=w226, "Value"="OK" ("值")) -> ()  [unwired: 1 in, 2 out]
                                n489 = call "Colour -ECU.vi"("result"="OK", "colourRef"=w225) -> ()  [unwired: 9 in, 1 out]
                                n490 = Wait (ms)(milliseconds to wait=u32 100 ("等待时间（毫秒）")) -> ()  [unwired: 1 out]
                              }
                              frame Default {
                                n491 = global read "Global1.vi" "ECU上序状态"() -> (w232:refnum<vi>)
                                n492 = Wait (ms)(milliseconds to wait=u32 2000 ("等待时间（毫秒）")) -> ()  [unwired: 1 out]
                                n493 = call "浮动通知2.vi"("通知内容"="ECU工位上序漏序！" ("Status")) -> ()  [unwired: 11 in]
                                n494 = global read "Global.vi" "ECU前序显示字"() -> (w229:refnum<vi>)
                                n495 = call "Colour.vi"("result"="等待", "colourRef"=w232) -> ()  [unwired: 9 in, 1 out]
                                n496 = shared-variable "我的电脑\\A17031611.lvlib\\设备状态2"(i16 6 ("设备状态控制字")) -> ()  [unwired: 1 in, 1 out]
                                n497 = property class="Str"(reference=w229, "Value"="漏序" ("值")) -> ()  [unwired: 1 in, 2 out]
                              }
                              frame "NG" {
                                n498 = Wait (ms)(milliseconds to wait=u32 2000 ("等待时间（毫秒）")) -> ()  [unwired: 1 out]
                                n499 = global read "Global1.vi" "ECU上序状态"() -> (w238:refnum<vi>)
                                n500 = call "浮动通知2.vi"("通知内容"="上序生产结果不合格！" ("Status")) -> ()  [unwired: 11 in]
                                n501 = global read "Global.vi" "ECU前序显示字"() -> (w240:refnum<vi>)
                                n502 = call "Colour -ECU.vi"("result"="NG", "colourRef"=w238) -> ()  [unwired: 9 in, 1 out]
                                n503 = shared-variable "我的电脑\\A17031611.lvlib\\设备状态2"(i16 6 ("设备状态控制字")) -> ()  [unwired: 1 in, 1 out]
                                n504 = property class="Str"(reference=w240, "Value"="NG" ("值")) -> ()  [unwired: 1 in, 2 out]
                              }
                            }
                          }
                        }
                      }
                    }
                  }
                  frame "exit" {
                  }
                }
                n505 = local write "STEP2"(w191) -> ()
              }
              frame #1 {
                n506 = Wait (ms)(milliseconds to wait=u32 100 ("等待时间（毫秒）")) -> ()  [unwired: 1 out]
              }
            }
          }
          frame "控制器扫码" {
            n507 = stacked-sequence {
              frame #0 {
                w247 = "请扫请控制器码！！" ("提示信息")
                n508 = call "输入框.vi"("提示信息"=w247) -> ("条形码输出"=w248:string)
                n509 = call "浮动通知2.vi"("通知内容"=w247) -> ()  [unwired: 11 in]
                n510 = case shown="\"\", 默认" w248 {
                  selector: w248 -> [w252 _]
                  tunnel: [w257 "手动"] -> w249
                  frame "", Default {
                    (unwired) "-" ("正则表达式")
                    n511 = global read "Global.vi" "硬件版本号"() -> (w253:string)
                    n512 = global write "Global1.vi" "控制器码"(w252) -> ()
                    n513 = shared-variable "我的电脑\\Global.lvlib\\控制器码"(w252) -> ()  [unwired: 1 in, 1 out]
                    n514 = String Subset "截取字符串"(string=w252, length (rest)=11 ("长度（剩余）")) -> (substring=w250:string)  [unwired: 1 in]
                    n515 = call <vilib>:"Trim Whitespace.vi"("string"=w250) -> ("trimmed string"=w255:string)  [unwired: 1 in]
                    n516 = call <vilib>:"Trim Whitespace.vi"("string"=w253) -> ("trimmed string"=w256:string)  [unwired: 1 in]
                    n517 = Equal?(x=w255, y=w256) -> (x = y?=w254:bool)
                    n518 = case shown="假" w254 {
                      tunnel: ["控制器扫码" ("State(s) in Front (\"\")") w263] -> w257
                      frame False {
                        w261 = 0 items=["OK", "OKCancel", "AbortRetryIgnore", "YesNoCancel", "YesNo", "RetryCancel"] ("buttons")
                        w262 = 16 items=["None"=0, "Hand, Error, Stop"=16, "Question"=32, "Exclamation, Warning"=48, "Asterisk, Information"=64] ("icon")
                        n519 = call "信息框（标题、文本、图标）.vi"("icon"=w262, "buttons"=w261, "caption"="控制器混料", "text"="混料请核对控制器!") -> ()  [unwired: 6 in, 2 out]
                      }
                      frame True {
                        n520 = global read "Global1.vi" "联机模式"() -> (w264:enum16{"单机", "联网"})
                        n521 = case shown="\"单机\", 默认" w264 {
                          tunnel: ["步骤" ("State(s) in Front (\"\")") "步骤"] -> w263
                          frame "单机", Default {
                            n522 = global read "Global.vi" "安装支架生产数量"() -> (w268:refnum<vi>)
                            n523 = property class="Num"(reference=w268) -> (reference out=w269:refnum<vi>, error out=w270:errorcluster, "Value"=w271:variant)  [unwired: 1 in]
                            n524 = Variant To Data(type=u32 0, Variant=w271) -> (data=w272:u32)  [unwired: 1 in, 1 out]
                            n525 = Increment(x=w272) -> (x+1=w273:u32)
                            n526 = property class="Num"(reference=w269, error in=w270, "Value"=w273) -> ()  [unwired: 2 out]
                            n527 = Wait (ms)(milliseconds to wait=u32 10 ("等待时间（毫秒）")) -> ()  [unwired: 1 out]
                          }
                          frame "联网" {
                            n528 = global read "Global.vi" "安装支架生产数量"() -> (w276:refnum<vi>)
                            n529 = property class="Num"(reference=w276) -> (reference out=w277:refnum<vi>, error out=w278:errorcluster, "Value"=w279:variant)  [unwired: 1 in]
                            n530 = Variant To Data "变体至数据转换"(type=u32 0, Variant=w279) -> (data=w280:u32)  [unwired: 1 in, 1 out]
                            n531 = Wait (ms)(milliseconds to wait=u32 100 ("等待时间（毫秒）")) -> ()  [unwired: 1 out]
                            n532 = Increment(x=w280) -> (x+1=w281:u32)
                            n533 = property class="Num"(reference=w277, error in=w278, "Value"=w281) -> ()  [unwired: 2 out]
                          }
                        }
                      }
                    }
                  }
                  frame "exit" {
                  }
                }
                n534 = local write "STEP2"(w249) -> ()
              }
              frame #1 {
                n535 = Wait (ms)(milliseconds to wait=u32 100 ("等待时间（毫秒）")) -> ()  [unwired: 1 out]
              }
            }
          }
          frame "自动" {
            # "3=41\n2=42\n1=43\n0=45"
            # "4=31\n3=32\n2=33\n1=34\n0=35"
            n536 = shared-variable "我的电脑\\A17031611.lvlib\\安装支架螺栓2"() -> (w285:u16)  [unwired: 1 in, 1 out]
            n537 = shared-variable "我的电脑\\A17031611.lvlib\\安装支架螺栓数"() -> (w286:u16)  [unwired: 1 in, 1 out]
            n538 = shared-variable "我的电脑\\A17031611.lvlib\\设备状态2"() -> (w287:i16)  [unwired: 1 in, 1 out]
            n539 = global read "A170316-11.vi" "安装支架LED"() -> (w288:refnum<vi>[])
            n540 = case shown="6" w287 {
              tunnel: w288 -> [_ _ _ _ _ w292 _ _ w304 w312 w316 w324 w328 w336 _ w340 w348 w352 w360 w364 w372 w376 w384 w389 w394 _ _ w406 w409 w416 _ _ w441 _ _ _ _]
              tunnel: w286 -> [_ _ _ _ _ _ _ _ _ _ _ _ _ _ _ _ _ _ _ _ _ _ _ _ _ _ _ _ _ _ _ _ _ _ _ _ _]
              tunnel: w285 -> [_ _ _ _ _ _ _ _ _ _ _ _ _ _ _ _ _ _ _ _ _ _ _ _ _ _ _ _ _ _ _ _ _ _ _ _ _]
              frame Default {
              }
              frame -128 {
                n541 = global read "Global.vi" "ECU自动"() -> (w290:refnum<vi>)
                n542 = property class="Bool (严格)"(reference=w290, "Value"=FALSE) -> ()  [unwired: 1 in, 2 out]
              }
              frame 5 {
                (unwired) "ECU工位复位完成！" ("Status")
              }
              frame 6 {
                n543 = call "浮动通知3.vi"("通知内容"="请按启动确认扫ECU工位主码") -> ()  [unwired: 11 in]
              }
              frame 0 {
                (unwired) "手动状态！" ("Status")
              }
              frame 7 {
                n544 = for {
                  tunnel: w292 -> [w299] mode=indexing
                  n545 = call "Colour -ECU.vi"("result"="", "colourRef"=w299) -> ()  [unwired: 9 in, 1 out]
                }
                n546 = global read "Global.vi" "ECU结果显示"() -> (w294:refnum<vi>)
                n547 = property class="Str"(reference=w294, "Value"="..." ("结果显示")) -> (reference out=w295:refnum<vi>)  [unwired: 1 in, 1 out]
                n548 = property class="Str"(reference=w295, "Text.TextColor"=u32 16776960) -> ()  [unwired: 1 in, 2 out]
                n549 = local write "STEP2"("扫主码" ("STEP2")) -> ()
              }
              frame 9 {
              }
              frame 10 {
                n550 = shared-variable "我的电脑\\A17031611.lvlib\\设备状态2"(i16 31 ("设备状态")) -> ()  [unwired: 1 in, 1 out]
              }
              frame 31 {
                n551 = Index Array(array=w304, index=0 ("索引")) -> (element=w303:refnum<vi>)
                n552 = call "Colour -ECU.vi"("result"="等待", "colourRef"=w303) -> ()  [unwired: 9 in, 1 out]
                n553 = call "浮动通知3.vi"("通知内容"="请安装固定螺栓1并确认扭矩！" ("Status")) -> ()  [unwired: 11 in]
              }
              frame 32 {
                n554 = Index Array(array=w312, index #1=0 ("索引"), index #2=1 ("索引")) -> (element #1=w311:refnum<vi>, element #2=w309:refnum<vi>)
                n555 = shared-variable "我的电脑\\A17031611.lvlib\\设备状态2"(i16 33 ("设备状态2")) -> ()  [unwired: 1 in, 1 out]
                n556 = call "Colour -ECU.vi"("result"="等待", "colourRef"=w309) -> ()  [unwired: 9 in, 1 out]
                n557 = call "Colour -ECU.vi"("result"="OK", "colourRef"=w311) -> ()  [unwired: 9 in, 1 out]
              }
              frame 33 {
                n558 = Index Array(array=w316, index=1 ("索引")) -> (element=w315:refnum<vi>)
                n559 = call "浮动通知2.vi"("通知内容"="控制器安装螺栓2拧紧确认！" ("Status")) -> ()  [unwired: 11 in]
                n560 = call "Colour -ECU.vi"("result"="等待", "colourRef"=w315) -> ()  [unwired: 9 in, 1 out]
              }
              frame 34 {
                n561 = Index Array(array=w324, index #1=1 ("索引")) -> (element #1=w323:refnum<vi>, element #2=w320:refnum<vi>)  [unwired: 1 in]
                n562 = shared-variable "我的电脑\\A17031611.lvlib\\设备状态2"(i16 35 ("设备状态2")) -> ()  [unwired: 1 in, 1 out]
                n563 = call "Colour -ECU.vi"("result"="OK", "colourRef"=w323) -> ()  [unwired: 9 in, 1 out]
                n564 = call "Colour -ECU.vi"("result"="等待", "colourRef"=w320) -> ()  [unwired: 9 in, 1 out]
              }
              frame 35 {
                n565 = Index Array(array=w328, index=2 ("索引")) -> (element=w327:refnum<vi>)
                n566 = call "浮动通知2.vi"("通知内容"="控制器安装螺栓3拧紧确认!") -> ()  [unwired: 11 in]
                n567 = call "Colour -ECU.vi"("result"="等待", "colourRef"=w327) -> ()  [unwired: 9 in, 1 out]
              }
              frame 36 {
                n568 = Index Array(array=w336, index #1=2 ("索引")) -> (element #1=w333:refnum<vi>, element #2=w332:refnum<vi>)  [unwired: 1 in]
                n569 = shared-variable "我的电脑\\A17031611.lvlib\\设备状态2"(i16 41 ("设备状态2")) -> ()  [unwired: 1 in, 1 out]
                n570 = call "Colour -ECU.vi"("result"="OK", "colourRef"=w333) -> ()  [unwired: 9 in, 1 out]
                n571 = call "Colour -ECU.vi"("result"="等待", "colourRef"=w332) -> ()  [unwired: 9 in, 1 out]
              }
              frame 40 {
              }
              frame 41 {
                n572 = Index Array(array=w340, index=3 ("索引")) -> (element=w339:refnum<vi>)
                n573 = call "浮动通知2.vi"("通知内容"="请安装控制器支架1并确认扭矩！" ("Status")) -> ()  [unwired: 11 in]
                n574 = call "Colour -ECU.vi"("result"="等待", "colourRef"=w339) -> ()  [unwired: 9 in, 1 out]
              }
              frame 42 {
                n575 = Index Array(array=w348, index #1=3 ("索引")) -> (element #1=w346:refnum<vi>, element #2=w344:refnum<vi>)  [unwired: 1 in]
                n576 = shared-variable "我的电脑\\A17031611.lvlib\\设备状态2"(i16 43 ("设备状态2")) -> ()  [unwired: 1 in, 1 out]
                n577 = call "Colour -ECU.vi"("result"="等待", "colourRef"=w344) -> ()  [unwired: 9 in, 1 out]
                n578 = call "Colour -ECU.vi"("result"="OK", "colourRef"=w346) -> ()  [unwired: 9 in, 1 out]
              }
              frame 43 {
                n579 = Index Array(array=w352, index=4 ("索引")) -> (element=w350:refnum<vi>)
                n580 = call "浮动通知2.vi"("通知内容"="请安装控制器支架2并确认扭矩！" ("Status")) -> ()  [unwired: 11 in]
                n581 = call "Colour -ECU.vi"("result"="等待", "colourRef"=w350) -> ()  [unwired: 9 in, 1 out]
              }
              frame 44 {
                n582 = Index Array(array=w360, index #1=4 ("索引")) -> (element #1=w358:refnum<vi>, element #2=w356:refnum<vi>)  [unwired: 1 in]
                n583 = shared-variable "我的电脑\\A17031611.lvlib\\设备状态2"(i16 45 ("设备状态2")) -> ()  [unwired: 1 in, 1 out]
                n584 = call "Colour -ECU.vi"("result"="等待", "colourRef"=w356) -> ()  [unwired: 9 in, 1 out]
                n585 = call "Colour -ECU.vi"("result"="OK", "colourRef"=w358) -> ()  [unwired: 9 in, 1 out]
              }
              frame 45 {
                n586 = Index Array(array=w364, index=5 ("索引")) -> (element=w362:refnum<vi>)
                n587 = call "浮动通知2.vi"("通知内容"="请安装控制器支架3并确认扭矩") -> ()  [unwired: 11 in]
                n588 = call "Colour -ECU.vi"("result"="等待", "colourRef"=w362) -> ()  [unwired: 9 in, 1 out]
              }
              frame 46 {
                n589 = Index Array(array=w372, index #1=5 ("索引")) -> (element #1=w370:refnum<vi>, element #2=w368:refnum<vi>)  [unwired: 1 in]
                n590 = shared-variable "我的电脑\\A17031611.lvlib\\设备状态2"(i16 47 ("设备状态2")) -> ()  [unwired: 1 in, 1 out]
                n591 = call "Colour -ECU.vi"("result"="等待", "colourRef"=w368) -> ()  [unwired: 9 in, 1 out]
                n592 = call "Colour -ECU.vi"("result"="OK", "colourRef"=w370) -> ()  [unwired: 9 in, 1 out]
              }
              frame 47 {
                n593 = Index Array(array=w376, index=6 ("索引")) -> (element=w375:refnum<vi>)
                n594 = call "浮动通知2.vi"("通知内容"="请安装控制器支架4并确认扭矩") -> ()  [unwired: 11 in]
                n595 = call "Colour -ECU.vi"("result"="等待", "colourRef"=w375) -> ()  [unwired: 9 in, 1 out]
              }
              frame 48 {
                n596 = Index Array(array=w384, index #1=6 ("索引")) -> (element #1=w383:refnum<vi>, element #2=w380:refnum<vi>)  [unwired: 1 in]
                n597 = shared-variable "我的电脑\\A17031611.lvlib\\设备状态2"(i16 60 ("设备状态2")) -> ()  [unwired: 1 in, 1 out]
                n598 = call "Colour -ECU.vi"("result"="等待", "colourRef"=w380) -> ()  [unwired: 9 in, 1 out]
                n599 = call "Colour -ECU.vi"("result"="OK", "colourRef"=w383) -> ()  [unwired: 9 in, 1 out]
              }
              frame 60 {
                n600 = Index Array(array=w389, index=7 ("索引")) -> (element=w386:refnum<vi>)
                n601 = call "浮动通知2.vi"("通知内容"="请取记号笔标记!") -> ()  [unwired: 11 in]
                n602 = call "Colour -ECU.vi"("result"="等待", "colourRef"=w386) -> ()  [unwired: 9 in, 1 out]
              }
              frame 61 {
                n603 = Index Array(array=w394, index=7 ("索引")) -> (element=w392:refnum<vi>)
                n604 = call "Colour.vi"("result"="OK", "colourRef"=w392) -> ()  [unwired: 9 in, 1 out]
                n605 = shared-variable "我的电脑\\A17031611.lvlib\\设备状态2"(i16 200 ("设备状态2")) -> ()  [unwired: 1 in, 1 out]
              }
              frame 70 {
                n606 = control-ref of="安装支架线卡扎带安装"() -> (w397:refnum<vi>)
                n607 = call "Colour -ECU.vi"("result"="等待", "colourRef"=w397) -> ()  [unwired: 9 in, 1 out]
                n608 = call "浮动通知2.vi"("通知内容"="请取轧带！" ("Status")) -> ()  [unwired: 11 in]
              }
              frame 81 {
                n609 = stacked-sequence {
                  frame #0 {
                    n610 = local read "ECU步骤"() -> (w400:T2)
                    n611 = control-ref of="安装支架线卡扎带安装"() -> (w403:refnum<vi>)
                    n612 = Increment(x=w400) -> (x+1=w399:T2)
                    n613 = local write "ECU步骤"(w399) -> ()
                    n614 = call "浮动通知2.vi"("通知内容"="完成！" ("Status")) -> ()  [unwired: 11 in]
                    n615 = call "Colour -ECU.vi"("result"="OK", "colourRef"=w403) -> ()  [unwired: 9 in, 1 out]
                  }
                  frame #1 {
                    n616 = Wait (ms)(milliseconds to wait=u32 50 ("等待时间（毫秒）")) -> ()  [unwired: 1 out]
                  }
                  frame #2 {
                    n617 = local write "STEP2"("步骤" ("STEP2")) -> ()
                  }
                }
              }
              frame 71 {
                n618 = Index Array(array=w406, index #1=8 ("索引")) -> ()  [unwired: 1 in, 2 out]
                n619 = shared-variable "我的电脑\\A17031611.lvlib\\设备状态2"(i16 200 ("设备状态")) -> ()  [unwired: 1 in, 1 out]
              }
              frame 91 {
                (unwired) "请安装电机扎带并取走工件！" ("Status")
                n620 = Index Array(array=w409, index #1=5 ("索引")) -> (element #1=w411:refnum<vi>, element #2=w410:refnum<vi>)  [unwired: 1 in]
                n621 = call "Colour.vi"("result"="OK", "colourRef"=w411) -> ()  [unwired: 9 in, 1 out]
                n622 = call "Colour.vi"("result"="等待", "colourRef"=w410) -> ()  [unwired: 9 in, 1 out]
                n623 = shared-variable "我的电脑\\A17031611.lvlib\\设备状态3"(i16 100 ("设备状态")) -> ()  [unwired: 1 in, 1 out]
              }
              frame 101 {
                (unwired) "完成！" ("Status")
                n624 = Index Array(array=w416, index #1=6 ("索引")) -> (element #1=w418:refnum<vi>, element #2=w417:refnum<vi>)  [unwired: 1 in]
                n625 = call "Colour.vi"("result"="OK", "colourRef"=w418) -> ()  [unwired: 9 in, 1 out]
                n626 = call "Colour.vi"("result"="等待", "colourRef"=w417) -> ()  [unwired: 9 in, 1 out]
                n627 = shared-variable "我的电脑\\A17031611.lvlib\\设备状态3"(i16 110 ("设备状态")) -> ()  [unwired: 1 in, 1 out]
              }
              frame 200 {
                n628 = global read "Global.vi" "检测结果"() -> (w432:refnum<vi>)
                n629 = global write "Global1.vi" "ECU工位生产结果"("OK" ("电机工位生产结果")) -> ()
                n630 = call "浮动通知2.vi"("通知内容"="产品合格！" ("Status")) -> ()  [unwired: 11 in]
                n631 = call "Colour.vi"("result"="OK", "colourRef"=w432) -> ()  [unwired: 9 in, 1 out]
                n632 = global read "Global.vi" "ECU结果显示"() -> (w430:refnum<vi>)
                n633 = property class="Str"(reference=w430, "Value"="OK" ("结果显示")) -> (reference out=w427:refnum<vi>)  [unwired: 1 in, 1 out]
                n634 = global read "Global1.vi" "联机模式"() -> (w424:enum16{"单机", "联网"})
                n635 = property class="Str"(reference=w427, "Text.TextColor"=u32 6618880) -> ()  [unwired: 1 in, 2 out]
                n636 = case shown="\"联网\"" w424 {
                  tunnel: ["初始化" "录入数据库" ("STEP3")] -> w423
                  frame "单机", Default {
                  }
                  frame "联网" {
                  }
                }
                n637 = local write "STEP2"(w423) -> ()
              }
              frame 201 {
                (unwired) "产品不合格！" ("Status")
                n638 = global read "Global.vi" "检测结果"() -> (w439:refnum<vi>)
                n639 = call "Colour.vi"("result"="NG", "colourRef"=w439) -> ()  [unwired: 9 in, 1 out]
                n640 = global read "Global.vi" "电机结果显示"() -> (w438:refnum<vi>)
                n641 = property class="Str"(reference=w438, "Value"="NG" ("结果显示")) -> (reference out=w437:refnum<vi>)  [unwired: 1 in, 1 out]
                n642 = property class="Str"(reference=w437, "Text.TextColor"=u32 16711680) -> ()  [unwired: 1 in, 2 out]
              }
              frame 999 {
                n643 = for {
                  tunnel: w441 -> [w444] mode=indexing
                  n644 = call "Colour.vi"("result"="", "colourRef"=w444) -> ()  [unwired: 9 in, 1 out]
                }
                n645 = call "浮动通知2.vi"("通知内容"="请重新安装固定螺栓！" ("Status")) -> ()  [unwired: 11 in]
                n646 = shared-variable "我的电脑\\A17031611.lvlib\\设备状态2"(i16 31 ("设备状态")) -> ()  [unwired: 1 in, 1 out]
              }
              frame 1024 {
                n647 = global read "Global.vi" "ECU自动"() -> (w447:refnum<vi>)
                n648 = property class="Bool (严格)"(reference=w447, "Value"=FALSE) -> ()  [unwired: 1 in, 2 out]
              }
              frame 3721 {
                (unwired) "产品不合格程序锁定！" ("Status")
                n649 = local write "STEP3"("不合格锁定" ("STEP")) -> ()
              }
              frame 3722 {
                n650 = global read "Global.vi" "ECU自动"() -> (w450:refnum<vi>)
                n651 = property class="Bool (严格)"(reference=w450, "Value"=FALSE) -> ()  [unwired: 1 in, 2 out]
              }
              frame 3723 {
                (unwired) "请取出不合格产品并摆放至不合格品区！" ("Status")
              }
            }
          }
          frame "录入数据库" {
            n652 = stacked-sequence {
              frame #0 {
                n653 = Get Date/Time String(date format (0)=enum16{"short", "long", "abbreviated"}."short" ("日期格式(0)"), want seconds? (F)=FALSE ("需要秒？(F)")) -> (date string=w460:string, time string=w461:string)  [unwired: 1 in]
                n654 = global read "Global1.vi" "DEVICE_ID_ECU"() -> (w464:string)
                n655 = global read "Global1.vi" "CODE_ID_ECU"() -> (w463:string)
                n656 = global read "Global1.vi" "ECU工位生产结果"() -> (w455:string)
                n657 = global read "Global1.vi" "USER_ID"() -> (w462:string)
                n658 = Concatenate Strings(w460, " " ("字符串"), w461) -> (w456:string)
                n659 = Decimal String To Number(string=w464, default (0L)=i64 0 ("默认(0 I32)")) -> (number=w453:i64)  [unwired: 1 in, 1 out]
                n660 = Decimal String To Number(string=w462, default (0L)=i64 0 ("默认(0 I32)")) -> (number=w452:i64)  [unwired: 1 in, 1 out]
                n661 = Decimal String To Number(string=w463, default (0L)=i64 0 ("默认(0 I32)")) -> (number=w451:i64)  [unwired: 1 in, 1 out]
                n662 = global read "Global1.vi" "联机模式"() -> (w471:enum16{"单机", "联网"})
                n663 = Search and Replace String(replace all?=TRUE ("替换全部？(F)"), input string=w456, search string="/" ("替换字符串(\"\")"), replace string="-" ("替换字符串(\"\")")) -> (result string=w454:string)  [unwired: 4 in, 3 out]
                n664 = Bundle(w453, w452, w451, "ECU工位生产结果"=w455, "result string"=w454) -> (w477:T8)  [unwired: 1 in]
                n665 = call "GetSQLstring.vi"("联机模式"=w471) -> ("错误输出"=w474:errorcluster, "连接字符串"=w473:string)  [unwired: 9 in]
                n666 = Build Array(w477) -> (w478:T9)
                n667 = call-poly <vilib>:"DB Tools Open Connection.vi"("error in (no error)"=w474, "connection information"=w473) -> ("error out"=w472:errorcluster, "connection reference"=w475:T6)  [unwired: 6 in]
                n668 = for {
                  tunnel: w478 -> [w483] mode=indexing
                  tunnel: w475 -> [w481]
                  shift-right: [w479] -> w476
                  shift-left: w472 -> [w486]
                  w482 = string[] ["DEVICE_ID", "USER_ID", "CODE_ID", "RESULT_VALUE", "RESULT_TIME"] ("columns")
                  w484 = "Result" ("table")
                  n669 = call <vilib>:"DB Tools Insert Data.vi"("data"=w483, "error in (no error)"=w486, "columns"=w482, "table"=w484, "connection reference"=w481) -> ("error out"=w485:errorcluster, "connection reference out"=w480:T6)  [unwired: 5 in]
                  n670 = case shown="错误" w485 {
                    selector: w485 -> [w487 w508]
                    tunnel: w482 -> [_ w505]
                    tunnel: w480 -> [w488 w497]
                    tunnel: w484 -> [_ w509]
                    tunnel: w483 -> [_ w501]
                    tunnel: [w488 w496] -> _
                    tunnel: [w487 w495] -> w479
                    frame No Error {
                    }
                    frame Error {
                      n671 = Array Subset(array=w505, index=3 ("长度"), length=2 ("长度")) -> (w506:string[])
                      n672 = Unbundle(w501) -> (w490:i64, w493:i64, "ECU工位生产结果"=w500:string, "result string"=w499:string)  [unwired: 1 out]
                      n673 = Number To Decimal String(number=w493) -> (decimal integer string=w494:string)  [unwired: 1 in]
                      n674 = Number To Decimal String(number=w490) -> (decimal integer string=w489:string)  [unwired: 1 in]
                      n675 = Concatenate Strings("WHERE CODE_ID =" ("condition"), w494, "AND DEVICE_ID = ", w489) -> (w502:string)
                      n676 = Bundle("ECU工位生产结果"=w500, "result string"=w499) -> (w498:T10)  [unwired: 1 in]
                      n677 = call <vilib>:"Clear Errors.vi"("error in (no error)"=w508) -> ("error out"=w507:errorcluster)  [unwired: 5 in, 1 out]
                      n678 = call <vilib>:"DB Tools Update Data.vi"("condition"=w502, "data"=w498, "error in (no error)"=w507, "columns"=w506, "table"=w509, "connection reference"=w497) -> ("error out"=w495:errorcluster, "connection reference out"=w496:T6)  [unwired: 4 in]
                    }
                  }
                }
                n679 = call <vilib>:"Simple Error Handler.vi"("error in (no error)"=w476) -> ()  [unwired: 4 in, 5 out]
              }
              frame #1 {
                n680 = global read "Global1.vi" "CODE_ID_ECU"() -> (w511:string)
                n681 = global read "Global1.vi" "控制器码"() -> (w510:string)
                n682 = Format Into String(format string="UPDATE\ndbo.[Code]\nSET dbo.[Code].CODE_ECU = '%s'\n\nWHERE\ndbo.[Code].CODE_ID = %s\n" ("格式字符串"), w510, w511) -> (resulting string=w514:string)  [unwired: 2 in, 1 out]
                n683 = call "SQL_query.vi"("SQL query"=w514, "联机模式"=enum16{"单机", "联网"}."联网") -> ()  [unwired: 1 in, 3 out]
              }
              frame #2 {
                n684 = call "浮动通知2.vi"("通知内容"="ECU工位数据录入成功！" ("Status")) -> ()  [unwired: 11 in]
                n685 = local write "STEP2"("初始化" ("STEP2")) -> ()
              }
            }
          }
          frame "步骤" {
            n686 = case shown="\"控制器安装螺栓1\", 默认" "ECU步骤" {
              selector: "ECU步骤" -> [w520 _]
              tunnel: [w519 "等待"] -> w517
              frame "控制器安装螺栓1", Default {
                n687 = global read "Global.vi" "控制器安装支架"() -> (w522:bool[])
                n688 = Index Array(array=w522, index=w520) -> (element=w521:bool)
                n689 = case shown="真" w521 {
                  tunnel: w520 -> [_ w528]
                  tunnel: ["步骤" w527] -> w519
                  frame False {
                    n690 = local read "ECU步骤"() -> (w526:T2)
                    n691 = Increment(x=w526) -> (x+1=w525:T2)
                    n692 = Wait (ms)(milliseconds to wait=u32 100 ("等待时间（毫秒）")) -> ()  [unwired: 1 out]
                    n693 = local write "ECU步骤"(w525) -> ()
                  }
                  frame True {
                    n694 = case shown="\"控制器安装螺栓2\"" w528 {
                      tunnel: ["等待" "等待" "等待" "等待" "等待" "等待" "等待" "等待" "等待"] -> w527
                      frame "控制器安装螺栓1", Default {
                        n695 = shared-variable "我的电脑\\A17031611.lvlib\\设备状态2"(i16 31 ("设备状态控制字")) -> ()  [unwired: 1 in, 1 out]
                      }
                      frame "控制器安装螺栓2" {
                        n696 = shared-variable "我的电脑\\A17031611.lvlib\\设备状态2"(i16 33 ("设备状态控制字")) -> ()  [unwired: 1 in, 1 out]
                      }
                      frame "控制器安装螺栓3" {
                        n697 = shared-variable "我的电脑\\A17031611.lvlib\\设备状态2"(i16 35 ("设备状态控制字")) -> ()  [unwired: 1 in, 1 out]
                      }
                      frame "安装支架螺栓1" {
                        n698 = shared-variable "我的电脑\\A17031611.lvlib\\设备状态2"(i16 41 ("设备状态控制字")) -> ()  [unwired: 1 in, 1 out]
                      }
                      frame "安装支架螺栓2" {
                        n699 = shared-variable "我的电脑\\A17031611.lvlib\\设备状态2"(i16 43 ("设备状态控制字")) -> ()  [unwired: 1 in, 1 out]
                      }
                      frame "安装支架螺栓3" {
                        n700 = shared-variable "我的电脑\\A17031611.lvlib\\设备状态2"(i16 45 ("设备状态控制字")) -> ()  [unwired: 1 in, 1 out]
                      }
                      frame "安装支架螺栓4" {
                        n701 = shared-variable "我的电脑\\A17031611.lvlib\\设备状态2"(i16 47 ("设备状态控制字")) -> ()  [unwired: 1 in, 1 out]
                      }
                      frame "涂色标" {
                        n702 = shared-variable "我的电脑\\A17031611.lvlib\\设备状态2"(i16 60 ("设备状态控制字")) -> ()  [unwired: 1 in, 1 out]
                      }
                      frame "安装线卡取走工件" {
                        n703 = shared-variable "我的电脑\\A17031611.lvlib\\设备状态2"(i16 70 ("设备状态控制字")) -> ()  [unwired: 1 in, 1 out]
                      }
                    }
                  }
                }
              }
              frame "完成" {
                n704 = shared-variable "我的电脑\\A17031611.lvlib\\设备状态2"(i16 200 ("设备状态控制字")) -> ()  [unwired: 1 in, 1 out]
              }
            }
            n705 = local write "STEP2"(w517) -> ()
          }
        }
        n706 = case shown="\"步骤\"" "STEP1" {
          frame "等待", Default {
            n707 = local write "STEP1"("自动" ("STEP1")) -> ()
            n708 = Wait (ms)(milliseconds to wait=u32 200 ("等待时间（毫秒）")) -> ()  [unwired: 1 out]
          }
          frame "初始化" {
            n709 = local write "STEP1"("步骤" ("STEP")) -> ()
            n710 = local write "控制器支架"(T1."控制器支架螺栓1" ("控制器支架")) -> ()
          }
          frame "自动" {
            # "5=31\n4=32\n3=33\n2=34\n1=35"
            n711 = shared-variable "我的电脑\\A17031611.lvlib\\控制器支架螺栓数量"() -> (w56:i16)  [unwired: 1 in, 1 out]
            n712 = shared-variable "我的电脑\\A17031611.lvlib\\设备状态1"() -> (w57:i16)  [unwired: 1 in, 1 out]
            n713 = global read "A170316-11.vi" "控制器支架LED"() -> (w58:refnum<vi>[])
            n714 = case shown="91" w57 {
              tunnel: w58 -> [_ _ _ _ _ _ _ _ _ _ _ _ _ w102 _ w112 w120 w135]
              tunnel: w56 -> [_ _ _ _ _ _ _ _ _ _ _ _ _ _ _ _ _ _]
              frame 0, Default {
              }
              frame 10 {
                n715 = local write "STEP1"("初始化" ("STEP1")) -> ()
              }
              frame 30 {
                n716 = control-ref of="控制器支架螺栓1拧紧确认"() -> (w60:refnum<vi>)
                n717 = call "Colour.vi"("result"="等待", "colourRef"=w60) -> ()  [unwired: 9 in, 1 out]
              }
              frame 31 {
                n718 = stacked-sequence {
                  frame #0 {
                    n719 = local read "控制器支架"() -> (w62:T1)
                    n720 = control-ref of="控制器支架螺栓1拧紧确认"() -> (w65:refnum<vi>)
                    n721 = Increment(x=w62) -> (x+1=w63:T1)
                    n722 = local write "控制器支架"(w63) -> ()
                    n723 = call "Colour.vi"("result"="OK", "colourRef"=w65) -> ()  [unwired: 9 in, 1 out]
                  }
                  frame #1 {
                    n724 = Wait (ms)(milliseconds to wait=u32 50 ("等待时间（毫秒）")) -> ()  [unwired: 1 out]
                  }
                  frame #2 {
                    n725 = local write "STEP1"("步骤" ("STEP1")) -> ()
                  }
                }
              }
              frame 32 {
                n726 = control-ref of="控制器支架螺栓2拧紧确认"() -> (w68:refnum<vi>)
                n727 = call "Colour.vi"("result"="等待", "colourRef"=w68) -> ()  [unwired: 9 in, 1 out]
              }
              frame 33 {
                n728 = stacked-sequence {
                  frame #0 {
                    n729 = local read "控制器支架"() -> (w70:T1)
                    n730 = control-ref of="控制器支架螺栓2拧紧确认"() -> (w72:refnum<vi>)
                    n731 = Increment(x=w70) -> (x+1=w71:T1)
                    n732 = local write "控制器支架"(w71) -> ()
                    n733 = call "Colour.vi"("result"="OK", "colourRef"=w72) -> ()  [unwired: 9 in, 1 out]
                  }
                  frame #1 {
                    n734 = Wait (ms)(milliseconds to wait=u32 50 ("等待时间（毫秒）")) -> ()  [unwired: 1 out]
                  }
                  frame #2 {
                    n735 = local write "STEP1"("步骤" ("STEP1")) -> ()
                  }
                }
              }
              frame 34 {
                # "控制器支架螺栓1"
                n736 = control-ref of="控制器支架螺栓3拧紧确认"() -> (w76:refnum<vi>)
                n737 = call "Colour.vi"("result"="等待", "colourRef"=w76) -> ()  [unwired: 9 in, 1 out]
              }
              frame 35 {
                n738 = stacked-sequence {
                  frame #0 {
                    n739 = control-ref of="控制器支架螺栓3拧紧确认"() -> (w80:refnum<vi>)
                    n740 = local read "控制器支架"() -> (w78:T1)
                    n741 = call "Colour.vi"("result"="OK", "colourRef"=w80) -> ()  [unwired: 9 in, 1 out]
                    n742 = Increment(x=w78) -> (x+1=w79:T1)
                    n743 = local write "控制器支架"(w79) -> ()
                  }
                  frame #1 {
                    n744 = Wait (ms)(milliseconds to wait=u32 50 ("等待时间（毫秒）")) -> ()  [unwired: 1 out]
                  }
                  frame #2 {
                    n745 = local write "STEP1"("步骤" ("STEP1")) -> ()
                  }
                }
              }
              frame 36 {
                n746 = control-ref of="控制器支架螺栓4拧紧确认"() -> (w84:refnum<vi>)
                n747 = call "Colour.vi"("result"="等待", "colourRef"=w84) -> ()  [unwired: 9 in, 1 out]
              }
              frame 37 {
                n748 = stacked-sequence {
                  frame #0 {
                    n749 = local read "控制器支架"() -> (w86:T1)
                    n750 = control-ref of="控制器支架螺栓4拧紧确认"() -> (w88:refnum<vi>)
                    n751 = Increment(x=w86) -> (x+1=w87:T1)
                    n752 = local write "控制器支架"(w87) -> ()
                    n753 = call "Colour.vi"("result"="OK", "colourRef"=w88) -> ()  [unwired: 9 in, 1 out]
                  }
                  frame #1 {
                    n754 = Wait (ms)(milliseconds to wait=u32 50 ("毫秒计时值")) -> ()  [unwired: 1 out]
                  }
                  frame #2 {
                    n755 = local write "STEP1"("步骤" ("STEP1")) -> ()
                  }
                }
              }
              frame 38 {
                n756 = control-ref of="控制器支架螺栓5拧紧确认"() -> (w92:refnum<vi>)
                n757 = call "Colour.vi"("result"="等待", "colourRef"=w92) -> ()  [unwired: 9 in, 1 out]
              }
              frame 39 {
                n758 = stacked-sequence {
                  frame #0 {
                    n759 = local read "控制器支架"() -> (w94:T1)
                    n760 = control-ref of="控制器支架螺栓5拧紧确认"() -> (w96:refnum<vi>)
                    n761 = Increment(x=w94) -> (x+1=w95:T1)
                    n762 = call "Colour.vi"("result"="OK", "colourRef"=w96) -> ()  [unwired: 9 in, 1 out]
                    n763 = local write "控制器支架"(w95) -> ()
                  }
                  frame #1 {
                    n764 = Wait (ms)(milliseconds to wait=u32 50 ("等待时间（毫秒）")) -> ()  [unwired: 1 out]
                  }
                  frame #2 {
                    n765 = local write "STEP1"("步骤" ("STEP1")) -> ()
                  }
                }
              }
              frame 60 {
                n766 = control-ref of="控制器支架涂色标"() -> (w100:refnum<vi>)
                n767 = call "Colour.vi"("result"="等待", "colourRef"=w100) -> ()  [unwired: 9 in, 1 out]
              }
              frame 61 {
                n768 = Index Array(array=w102, index #1=4 ("索引")) -> ()  [unwired: 1 in, 2 out]
                n769 = stacked-sequence {
                  frame #0 {
                    n770 = local read "控制器支架"() -> (w104:T1)
                    n771 = control-ref of="控制器支架涂色标"() -> (w107:refnum<vi>)
                    n772 = Increment(x=w104) -> (x+1=w105:T1)
                    n773 = call "Colour.vi"("result"="OK", "colourRef"=w107) -> ()  [unwired: 9 in, 1 out]
                    n774 = local write "控制器支架"(w105) -> ()
                  }
                  frame #1 {
                    n775 = Wait (ms)(milliseconds to wait=u32 50 ("等待时间（毫秒）")) -> ()  [unwired: 1 out]
                  }
                  frame #2 {
                    n776 = local write "STEP1"("步骤" ("STEP1")) -> ()
                  }
                }
              }
              frame 70 {
                n777 = control-ref of="控制器支架安装线卡扎带"() -> (w110:refnum<vi>)
                n778 = call "Colour.vi"("result"="等待", "colourRef"=w110) -> ()  [unwired: 9 in, 1 out]
              }
              frame 81 {
                n779 = Index Array(array=w112, index=6 ("索引")) -> ()  [unwired: 1 out]
                n780 = stacked-sequence {
                  frame #0 {
                    n781 = local read "控制器支架"() -> (w114:T1)
                    n782 = control-ref of="控制器支架安装线卡扎带"() -> (w117:refnum<vi>)
                    n783 = Increment(x=w114) -> (x+1=w115:T1)
                    n784 = call "Colour.vi"("result"="OK", "colourRef"=w117) -> ()  [unwired: 9 in, 1 out]
                    n785 = local write "控制器支架"(w115) -> ()
                  }
                  frame #1 {
                    n786 = Wait (ms)(milliseconds to wait=u32 50 ("毫秒计时值")) -> ()  [unwired: 1 out]
                  }
                  frame #2 {
                    n787 = local write "STEP1"("步骤" ("STEP1")) -> ()
                  }
                }
              }
              frame 91 {
                n788 = for {
                  tunnel: w120 -> [w123] mode=indexing
                  n789 = call "Colour.vi"("result"="", "colourRef"=w123) -> ()  [unwired: 9 in, 1 out]
                }
                n790 = shared-variable "我的电脑\\A17031611.lvlib\\设备状态1"(i16 8 ("设备状态")) -> ()  [unwired: 1 in, 1 out]
                n791 = call "浮动通知2.vi"("通知内容"="控制器和支架合装完成！" ("Status")) -> ()  [unwired: 11 in]
              }
              frame 999 {
                n792 = Index Array(array=w135, index #1=0 ("索引")) -> (element #1=w138:refnum<vi>, element #2=w132:refnum<vi>, element #3=w130:refnum<vi>, element #4=w128:refnum<vi>, element #5=w125:refnum<vi>)  [unwired: 4 in]
                n793 = call "Colour.vi"("result"="", "colourRef"=w125) -> ()  [unwired: 9 in, 1 out]
                n794 = call "Colour.vi"("result"="", "colourRef"=w132) -> ()  [unwired: 9 in, 1 out]
                n795 = call "Colour.vi"("result"="", "colourRef"=w130) -> ()  [unwired: 9 in, 1 out]
                n796 = call "Colour.vi"("result"="", "colourRef"=w128) -> ()  [unwired: 9 in, 1 out]
                n797 = call "Colour.vi"("result"="NG", "colourRef"=w138) -> ()  [unwired: 9 in, 1 out]
                n798 = call "浮动通知2.vi"("通知内容"="安装固定螺栓未完成，请重新安装！" ("Status")) -> ()  [unwired: 11 in]
                n799 = shared-variable "我的电脑\\A17031611.lvlib\\设备状态1"(i16 10 ("设备状态")) -> ()  [unwired: 1 in, 1 out]
              }
            }
          }
          frame "步骤" {
            n800 = case shown="\"完成\"" "控制器支架" {
              selector: "控制器支架" -> [w142 _]
              tunnel: [w141 "等待"] -> w139
              frame "控制器支架螺栓1", Default {
                n801 = global read "Global.vi" "控制器支架"() -> (w144:bool[])
                n802 = Index Array(array=w144, index=w142) -> (element=w143:bool)
                n803 = case shown="真" w143 {
                  tunnel: w142 -> [_ w149]
                  tunnel: ["步骤" w148] -> w141
                  frame False {
                    n804 = local read "控制器支架"() -> (w147:T1)
                    n805 = Increment(x=w147) -> (x+1=w146:T1)
                    n806 = local write "控制器支架"(w146) -> ()
                  }
                  frame True {
                    n807 = case shown="\"安装线卡轧带\"" w149 {
                      tunnel: ["等待" "等待" "等待" "等待" "等待" "等待" "等待"] -> w148
                      frame "控制器支架螺栓1", Default {
                        n808 = shared-variable "我的电脑\\A17031611.lvlib\\设备状态1"(i16 30 ("设备状态1")) -> ()  [unwired: 1 in, 1 out]
                      }
                      frame "控制器支架螺栓2" {
                        n809 = shared-variable "我的电脑\\A17031611.lvlib\\设备状态1"(i16 32 ("设备状态1")) -> ()  [unwired: 1 in, 1 out]
                      }
                      frame "控制器支架螺栓3" {
                        n810 = shared-variable "我的电脑\\A17031611.lvlib\\设备状态1"(i16 34 ("设备状态1")) -> ()  [unwired: 1 in, 1 out]
                      }
                      frame "控制器支架螺栓4" {
                        n811 = shared-variable "我的电脑\\A17031611.lvlib\\设备状态1"(i16 36 ("设备状态1")) -> ()  [unwired: 1 in, 1 out]
                      }
                      frame "控制器支架螺栓5" {
                        n812 = shared-variable "我的电脑\\A17031611.lvlib\\设备状态1"(i16 38 ("设备状态1")) -> ()  [unwired: 1 in, 1 out]
                      }
                      frame "涂色标" {
                        n813 = shared-variable "我的电脑\\A17031611.lvlib\\设备状态1"(i16 60 ("设备状态1")) -> ()  [unwired: 1 in, 1 out]
                      }
                      frame "安装线卡轧带" {
                        n814 = shared-variable "我的电脑\\A17031611.lvlib\\设备状态1"(i16 70 ("设备状态1")) -> ()  [unwired: 1 in, 1 out]
                      }
                    }
                  }
                }
              }
              frame "完成" {
                n815 = shared-variable "我的电脑\\A17031611.lvlib\\设备状态1"(i16 91 ("设备状态")) -> ()  [unwired: 1 in, 1 out]
              }
            }
            n816 = local write "STEP1"(w139) -> ()
          }
        }
        n817 = global read "Global.vi" "程序关闭"() -> (w48:bool)
      }
      n818 = while {
        stop <- w1078 stop-if-true
        n819 = global read "Global.vi" "产品型号"() -> (w1079:string)
        n820 = call "Is Value Changed.vim"("value"=w1079) -> ("changed or first call?"=w1080:bool)
        n821 = event shown="[2] \"更换产品\": 值改变" {
          selector: _ -> [_ _ _ _]
          dyn-events: _ -> [_ _ _ _]
          timeout: 5 -> [_ _ _ _]
          tunnel: w1079 -> [_ w1099 w1385 _]
          event Timeout {
            n822 = event-data() -> ()  [unwired: 1 in, 3 out]
            n823 = shared-variable "我的电脑\\A17031611.lvlib\\错误代码"() -> (w1083:u16)  [unwired: 1 in, 1 out]
            n824 = feedback #1() -> (w1093:u16)  [unwired: 1 in]
            n825 = feedback-in #1(w1083) -> ()
            n826 = Greater Or Equal?(x=w1083, y=i16 5000) -> (x >= y?=w1091:bool)
            n827 = Less?(x=w1083, y=i16 5200) -> (x < y?=w1092:bool)
            n828 = Equal?(x=w1083, y=w1093) -> (x = y?=w1090:bool)
            n829 = global read "Global.vi" "报警图标"() -> (w1085:refnum<vi>)
            n830 = And(x=w1091, y=w1092) -> (x .and. y?=w1084:bool)
            n831 = property class="Bool"(reference=w1085, "Value"=w1084) -> ()  [unwired: 1 in, 2 out]
            n832 = Bundle By Name(cluster=errorcluster {"status"=FALSE, "code"=0, "source"=""} ("错误常量"), "status"=w1084, "code"=w1083) -> (w1089:errorcluster)
            n833 = case shown="真" w1090 {
              tunnel: w1089 -> [w1098 _]
              frame False {
                n834 = call "报警处理.vi"("错误常量"=w1098) -> ()  [unwired: 9 in, 2 out]
              }
              frame True {
              }
            }
            n835 = case shown="0" w1083 {
              frame 0 {
                n836 = global read "Global.vi" "报警图标"() -> (w1094:refnum<vi>)
                n837 = property class="Bool"(reference=w1094, "Visible"=FALSE ("可见")) -> ()  [unwired: 1 in, 2 out]
              }
              frame 1, Default {
                n838 = global read "Global.vi" "报警图标"() -> (w1097:refnum<vi>)
                n839 = property class="Bool"(reference=w1097, "Visible"=TRUE ("可见")) -> ()  [unwired: 1 in, 2 out]
              }
            }
          }
          event "前序OK？": Value Change {
            n840 = event-data() -> ()  [unwired: 1 in, 6 out]
            n841 = stacked-sequence {
              tunnel: w1099 -> [_ w1153]
              frame #0 {
                n842 = disable-structure shown="禁用" {
                  frame Disabled {
                    n843 = control-ref of="安装扎带并取走工件"() -> (w1106:refnum<vi>)
                    n844 = control-ref of="安装扎带和线卡并取走工件"() -> (w1105:refnum<vi>)
                    n845 = control-ref of="控制器安装螺栓1拧紧确认"() -> (w1126:refnum<vi>)
                    n846 = control-ref of="控制器安装螺栓2拧紧确认"() -> (w1123:refnum<vi>)
                    n847 = control-ref of="安装支架涂色标"() -> (w1125:refnum<vi>)
                    n848 = control-ref of="安装支架扎带安装"() -> (w1109:refnum<vi>)
                    n849 = control-ref of="安装支架线卡扎带安装"() -> (w1108:refnum<vi>)
                    n850 = control-ref of="控制器安装螺栓3拧紧确认"() -> (w1104:refnum<vi>)
                    n851 = control-ref of="安装支架螺栓1拧紧确认"() -> (w1128:refnum<vi>)
                    n852 = control-ref of="安装支架螺栓4拧紧确认"() -> (w1100:refnum<vi>)
                    n853 = control-ref of="安装弹性垫圈并按启动拍照"() -> (w1115:refnum<vi>)
                    n854 = control-ref of="安装扎带并取走工件"() -> (w1110:refnum<vi>)
                    n855 = control-ref of="电机预拧紧螺栓2"() -> (w1113:refnum<vi>)
                    n856 = control-ref of="安装支架螺栓3拧紧确认"() -> (w1103:refnum<vi>)
                    n857 = control-ref of="安装支架螺栓2拧紧确认"() -> (w1127:refnum<vi>)
                    n858 = control-ref of="电机安装螺栓1扭矩确认"() -> (w1101:refnum<vi>)
                    n859 = control-ref of="按启动按钮拍照确认"() -> (w1112:refnum<vi>)
                    n860 = control-ref of="电机预拧紧螺栓1"() -> (w1114:refnum<vi>)
                    n861 = control-ref of="控制器支架涂色标"() -> (w1117:refnum<vi>)
                    n862 = control-ref of="涂色标"() -> (w1111:refnum<vi>)
                    n863 = Build Array(w1128, w1127, w1126, w1123, w1125, w1109, w1108, w1104, w1103, w1100) -> (w1124:refnum<vi>[])
                    n864 = control-ref of="控制器支架螺栓1拧紧确认"() -> (w1121:refnum<vi>)
                    n865 = control-ref of="控制器支架螺栓3拧紧确认"() -> (w1119:refnum<vi>)
                    n866 = for {
                      tunnel: w1124 -> [w1152] mode=indexing
                      i -> [w1151]
                      n867 = Multiply(x=60, y=w1151) -> (x*y=w1146:i32)
                      n868 = Add(x=340 ("y"), y=w1146) -> (x+y=w1148:i32)
                      n869 = Bundle("y"=-500, w1148) -> (w1147:cluster{"y":i32, i32})  [unwired: 1 in]
                      n870 = property class="Bool (严格)"(reference=w1152, "Position"=w1147) -> ()  [unwired: 1 in, 2 out]
                    }
                    n871 = control-ref of="控制器支架安装线卡扎带"() -> (w1107:refnum<vi>)
                    n872 = control-ref of="控制器支架螺栓4拧紧确认"() -> (w1118:refnum<vi>)
                    n873 = Build Array(w1115, w1114, w1113, w1112, w1111, w1110, w1106, w1105, w1101) -> (w1116:refnum<vi>[])
                    n874 = control-ref of="控制器支架螺栓2拧紧确认"() -> (w1120:refnum<vi>)
                    n875 = control-ref of="控制器支架螺栓5拧紧确认"() -> (w1102:refnum<vi>)
                    n876 = for {
                      tunnel: w1116 -> [w1136] mode=indexing
                      i -> [w1135]
                      n877 = Multiply(x=60, y=w1135) -> (x*y=w1133:i32)
                      n878 = Add(x=w1133, y=340) -> (x+y=w1130:i32)
                      n879 = Bundle("y"=-1500, w1130) -> (w1129:cluster{"y":i32, i32})  [unwired: 1 in]
                      n880 = property class="Bool (严格)"(reference=w1136, "Position"=w1129) -> ()  [unwired: 1 in, 2 out]
                    }
                    n881 = Build Array(w1121, w1120, w1119, w1118, w1117, w1107, w1102) -> (w1122:refnum<vi>[])
                    n882 = for {
                      tunnel: w1122 -> [w1144] mode=indexing
                      i -> [w1143]
                      n883 = Multiply(x=60, y=w1143) -> (x*y=w1141:i32)
                      n884 = Add(x=w1141, y=345) -> (x+y=w1138:i32)
                      n885 = Bundle("y"=-1000, w1138) -> (w1137:cluster{"y":i32, i32})  [unwired: 1 in]
                      n886 = property class="Bool (严格)"(reference=w1144, "Position"=w1137) -> ()  [unwired: 1 in, 2 out]
                    }
                  }
                  frame Enabled {
                  }
                }
              }
              frame #1 {
                n887 = disable-structure shown="禁用" {
                  disable-tunnel: w1153 -> [w1154 _]
                  frame Disabled {
                    n888 = case shown="\"R092B\"" w1154 {
                      frame Default {
                      }
                      frame "R92A" {
                        n889 = control-ref of="控制器安装螺栓2拧紧确认"() -> (w1159:refnum<vi>)
                        n890 = control-ref of="安装支架螺栓4拧紧确认"() -> (w1161:refnum<vi>)
                        n891 = control-ref of="控制器安装螺栓1拧紧确认"() -> (w1160:refnum<vi>)
                        n892 = control-ref of="安装支架螺栓1拧紧确认"() -> (w1164:refnum<vi>)
                        n893 = control-ref of="安装支架螺栓3拧紧确认"() -> (w1162:refnum<vi>)
                        n894 = control-ref of="控制器安装螺栓3拧紧确认"() -> (w1158:refnum<vi>)
                        n895 = control-ref of="安装支架涂色标"() -> (w1157:refnum<vi>)
                        n896 = control-ref of="安装支架螺栓2拧紧确认"() -> (w1163:refnum<vi>)
                        n897 = control-ref of="安装弹性垫圈并按启动拍照"() -> (w1171:refnum<vi>)
                        n898 = control-ref of="电机安装螺栓1扭矩确认"() -> (w1165:refnum<vi>)
                        n899 = control-ref of="电机预拧紧螺栓1"() -> (w1170:refnum<vi>)
                        n900 = control-ref of="电机预拧紧螺栓2"() -> (w1169:refnum<vi>)
                        n901 = control-ref of="按启动按钮拍照确认"() -> (w1168:refnum<vi>)
                        n902 = control-ref of="安装扎带并取走工件"() -> (w1166:refnum<vi>)
                        n903 = Build Array(w1164, w1163, w1162, w1161, w1160, w1159, w1158, w1157) -> (w1156:refnum<vi>[])
                        n904 = control-ref of="涂色标"() -> (w1167:refnum<vi>)
                        n905 = for {
                          tunnel: w1156 -> [w1201] mode=indexing
                          i -> [w1200]
                          n906 = Multiply(x=60, y=w1200) -> (x*y=w1195:i32)
                          n907 = Add(x=340 ("y"), y=w1195) -> (x+y=w1197:i32)
                          n908 = Bundle("y"=1775, w1197) -> (w1196:cluster{"y":i32, i32})  [unwired: 1 in]
                          n909 = property class="Bool (严格)"(reference=w1201, "Position"=w1196) -> ()  [unwired: 1 in, 2 out]
                        }
                        n910 = Build Array(w1171, w1170, w1169, w1165, w1168, w1167, w1166) -> (w1172:refnum<vi>[])
                        n911 = control-ref of="控制器支架螺栓2拧紧确认"() -> (w1175:refnum<vi>)
                        n912 = control-ref of="控制器支架螺栓1拧紧确认"() -> (w1176:refnum<vi>)
                        n913 = control-ref of="控制器支架螺栓3拧紧确认"() -> (w1174:refnum<vi>)
                        n914 = control-ref of="控制器支架螺栓4拧紧确认"() -> (w1173:refnum<vi>)
                        n915 = control-ref of="控制器支架涂色标"() -> (w1155:refnum<vi>)
                        n916 = for {
                          tunnel: w1172 -> [w1185] mode=indexing
                          i -> [w1184]
                          n917 = Multiply(x=60, y=w1184) -> (x*y=w1182:i32)
                          n918 = Add(x=w1182, y=340) -> (x+y=w1179:i32)
                          n919 = Bundle("y"=2115, w1179) -> (w1178:cluster{"y":i32, i32})  [unwired: 1 in]
                          n920 = property class="Bool (严格)"(reference=w1185, "Position"=w1178) -> ()  [unwired: 1 in, 2 out]
                        }
                        n921 = Build Array(w1176, w1175, w1174, w1173, w1155) -> (w1177:refnum<vi>[])
                        n922 = for {
                          tunnel: w1177 -> [w1193] mode=indexing
                          i -> [w1192]
                          n923 = Multiply(x=60, y=w1192) -> (x*y=w1190:i32)
                          n924 = Add(x=w1190, y=345) -> (x+y=w1187:i32)
                          n925 = Bundle("y"=1445, w1187) -> (w1186:cluster{"y":i32, i32})  [unwired: 1 in]
                          n926 = property class="Bool (严格)"(reference=w1193, "Position"=w1186) -> ()  [unwired: 1 in, 2 out]
                        }
                      }
                      frame "R128" {
                        # "1345"
                        n927 = control-ref of="安装支架螺栓2拧紧确认"() -> (w1217:refnum<vi>)
                        n928 = control-ref of="安装支架涂色标"() -> (w1216:refnum<vi>)
                        n929 = control-ref of="安装支架螺栓1拧紧确认"() -> (w1218:refnum<vi>)
                        n930 = control-ref of="控制器安装螺栓1拧紧确认"() -> (w1220:refnum<vi>)
                        n931 = control-ref of="控制器安装螺栓2拧紧确认"() -> (w1219:refnum<vi>)
                        n932 = control-ref of="安装弹性垫圈并按启动拍照"() -> (w1211:refnum<vi>)
                        n933 = control-ref of="电机预拧紧螺栓1"() -> (w1210:refnum<vi>)
                        n934 = control-ref of="电机预拧紧螺栓2"() -> (w1209:refnum<vi>)
                        n935 = control-ref of="涂色标"() -> (w1207:refnum<vi>)
                        n936 = control-ref of="安装扎带并取走工件"() -> (w1206:refnum<vi>)
                        n937 = control-ref of="按启动按钮拍照确认"() -> (w1208:refnum<vi>)
                        n938 = Build Array(w1220, w1219, w1218, w1217, w1216) -> (w1223:refnum<vi>[])
                        n939 = control-ref of="控制器支架螺栓2拧紧确认"() -> (w1214:refnum<vi>)
                        n940 = control-ref of="控制器支架螺栓1拧紧确认"() -> (w1215:refnum<vi>)
                        n941 = control-ref of="控制器支架螺栓3拧紧确认"() -> (w1213:refnum<vi>)
                        n942 = control-ref of="控制器支架螺栓5拧紧确认"() -> ()  [unwired: 1 out]
                        n943 = control-ref of="控制器支架涂色标"() -> (w1205:refnum<vi>)
                        n944 = control-ref of="控制器支架螺栓4拧紧确认"() -> (w1212:refnum<vi>)
                        n945 = for {
                          tunnel: w1223 -> [w1255] mode=indexing
                          i -> [w1254]
                          n946 = Multiply(x=60, y=w1254) -> (x*y=w1249:i32)
                          n947 = Add(x=438 ("y"), y=w1249) -> (x+y=w1251:i32)
                          n948 = Bundle("y"=-1495, w1251) -> (w1250:cluster{"y":i32, i32})  [unwired: 1 in]
                          n949 = property class="Bool (严格)"(reference=w1255, "Position"=w1250) -> ()  [unwired: 1 in, 2 out]
                        }
                        n950 = Build Array(w1211, w1210, w1209, w1208, w1207, w1206) -> (w1221:refnum<vi>[])
                        n951 = for {
                          tunnel: w1221 -> [w1239] mode=indexing
                          i -> [w1238]
                          n952 = Multiply(x=60, y=w1238) -> (x*y=w1236:i32)
                          n953 = Add(x=w1236, y=438) -> (x+y=w1233:i32)
                          n954 = Bundle("y"=-1145, w1233) -> (w1232:cluster{"y":i32, i32})  [unwired: 1 in]
                          n955 = property class="Bool (严格)"(reference=w1239, "Position"=w1232) -> ()  [unwired: 1 in, 2 out]
                        }
                        n956 = control-ref of="安装支架螺栓3拧紧确认"() -> (w1204:refnum<vi>)
                        n957 = Build Array(w1215, w1214, w1213, w1212, w1205) -> (w1222:refnum<vi>[])
                        n958 = control-ref of="安装支架螺栓4拧紧确认"() -> (w1202:refnum<vi>)
                        n959 = for {
                          tunnel: w1222 -> [w1247] mode=indexing
                          i -> [w1246]
                          n960 = Multiply(x=60, y=w1246) -> (x*y=w1244:i32)
                          n961 = Add(x=w1244, y=438) -> (x+y=w1241:i32)
                          n962 = Bundle("y"=-1820, w1241) -> (w1240:cluster{"y":i32, i32})  [unwired: 1 in]
                          n963 = property class="Bool (严格)"(reference=w1247, "Position"=w1240) -> ()  [unwired: 1 in, 2 out]
                        }
                        n964 = Build Array(w1204, w1202) -> (w1203:refnum<vi>[])
                        n965 = for {
                          tunnel: w1203 -> [w1231] mode=indexing
                          i -> [w1230]
                          n966 = Multiply(x=60, y=w1230) -> (x*y=w1228:i32)
                          n967 = Add(x=w1228, y=438) -> (x+y=w1225:i32)
                          n968 = Bundle("y"=-100, w1225) -> (w1224:cluster{"y":i32, i32})  [unwired: 1 in]
                          n969 = property class="Bool (严格)"(reference=w1231, "Position"=w1224) -> ()  [unwired: 1 in, 2 out]
                        }
                      }
                      frame "R092B" {
                        # "1345"
                        n970 = control-ref of="安装支架螺栓3拧紧确认"() -> (w1256:refnum<vi>)
                        n971 = control-ref of="安装支架涂色标"() -> (w1268:refnum<vi>)
                        n972 = control-ref of="安装支架螺栓2拧紧确认"() -> (w1269:refnum<vi>)
                        n973 = control-ref of="安装支架螺栓1拧紧确认"() -> (w1270:refnum<vi>)
                        n974 = control-ref of="控制器安装螺栓1拧紧确认"() -> (w1272:refnum<vi>)
                        n975 = control-ref of="控制器安装螺栓2拧紧确认"() -> (w1271:refnum<vi>)
                        n976 = control-ref of="安装弹性垫圈并按启动拍照"() -> (w1263:refnum<vi>)
                        n977 = control-ref of="电机预拧紧螺栓1"() -> (w1262:refnum<vi>)
                        n978 = control-ref of="电机预拧紧螺栓2"() -> (w1261:refnum<vi>)
                        n979 = control-ref of="涂色标"() -> (w1259:refnum<vi>)
                        n980 = control-ref of="安装扎带并取走工件"() -> (w1258:refnum<vi>)
                        n981 = control-ref of="按启动按钮拍照确认"() -> (w1260:refnum<vi>)
                        n982 = Build Array(w1272, w1271, w1270, w1269, w1256, w1268) -> (w1275:refnum<vi>[])
                        n983 = control-ref of="控制器支架螺栓2拧紧确认"() -> (w1266:refnum<vi>)
                        n984 = control-ref of="控制器支架螺栓1拧紧确认"() -> (w1267:refnum<vi>)
                        n985 = control-ref of="控制器支架螺栓3拧紧确认"() -> (w1265:refnum<vi>)
                        n986 = control-ref of="控制器支架涂色标"() -> (w1257:refnum<vi>)
                        n987 = control-ref of="控制器支架螺栓4拧紧确认"() -> (w1264:refnum<vi>)
                        n988 = for {
                          tunnel: w1275 -> [w1299] mode=indexing
                          i -> [w1298]
                          n989 = Multiply(x=60, y=w1298) -> (x*y=w1293:i32)
                          n990 = Add(x=438 ("y"), y=w1293) -> (x+y=w1295:i32)
                          n991 = Bundle("y"=-1495, w1295) -> (w1294:cluster{"y":i32, i32})  [unwired: 1 in]
                          n992 = property class="Bool (严格)"(reference=w1299, "Position"=w1294) -> ()  [unwired: 1 in, 2 out]
                        }
                        n993 = Build Array(w1263, w1262, w1261, w1260, w1259, w1258) -> (w1273:refnum<vi>[])
                        n994 = for {
                          tunnel: w1273 -> [w1283] mode=indexing
                          i -> [w1282]
                          n995 = Multiply(x=60, y=w1282) -> (x*y=w1280:i32)
                          n996 = Add(x=w1280, y=438) -> (x+y=w1277:i32)
                          n997 = Bundle("y"=-1145, w1277) -> (w1276:cluster{"y":i32, i32})  [unwired: 1 in]
                          n998 = property class="Bool (严格)"(reference=w1283, "Position"=w1276) -> ()  [unwired: 1 in, 2 out]
                        }
                        n999 = Build Array(w1267, w1266, w1265, w1264, w1257) -> (w1274:refnum<vi>[])
                        n1000 = control-ref of="控制器支架螺栓5拧紧确认"() -> ()  [unwired: 1 out]
                        n1001 = for {
                          tunnel: w1274 -> [w1291] mode=indexing
                          i -> [w1290]
                          n1002 = Multiply(x=60, y=w1290) -> (x*y=w1288:i32)
                          n1003 = Add(x=w1288, y=438) -> (x+y=w1285:i32)
                          n1004 = Bundle("y"=-1820, w1285) -> (w1284:cluster{"y":i32, i32})  [unwired: 1 in]
                          n1005 = property class="Bool (严格)"(reference=w1291, "Position"=w1284) -> ()  [unwired: 1 in, 2 out]
                        }
                      }
                      frame "R563X" {
                        # "1345"
                        n1006 = control-ref of="安装支架螺栓2拧紧确认"() -> (w1319:refnum<vi>)
                        n1007 = control-ref of="安装支架涂色标"() -> (w1318:refnum<vi>)
                        n1008 = control-ref of="安装支架螺栓1拧紧确认"() -> (w1320:refnum<vi>)
                        n1009 = control-ref of="控制器安装螺栓1拧紧确认"() -> (w1322:refnum<vi>)
                        n1010 = control-ref of="控制器安装螺栓2拧紧确认"() -> (w1321:refnum<vi>)
                        n1011 = control-ref of="安装弹性垫圈并按启动拍照"() -> (w1314:refnum<vi>)
                        n1012 = control-ref of="电机预拧紧螺栓1"() -> (w1313:refnum<vi>)
                        n1013 = control-ref of="电机预拧紧螺栓2"() -> (w1312:refnum<vi>)
                        n1014 = control-ref of="涂色标"() -> (w1310:refnum<vi>)
                        n1015 = control-ref of="安装扎带并取走工件"() -> (w1309:refnum<vi>)
                        n1016 = control-ref of="按启动按钮拍照确认"() -> (w1311:refnum<vi>)
                        n1017 = control-ref of="控制器支架螺栓2拧紧确认"() -> (w1316:refnum<vi>)
                        n1018 = control-ref of="控制器支架螺栓1拧紧确认"() -> (w1317:refnum<vi>)
                        n1019 = control-ref of="控制器支架螺栓3拧紧确认"() -> (w1315:refnum<vi>)
                        n1020 = control-ref of="控制器支架涂色标"() -> (w1308:refnum<vi>)
                        n1021 = Build Array(w1322, w1321, w1320, w1319, w1318) -> (w1325:refnum<vi>[])
                        n1022 = control-ref of="控制器支架螺栓5拧紧确认"() -> (w1303:refnum<vi>)
                        n1023 = control-ref of="控制器支架螺栓4拧紧确认"() -> (w1302:refnum<vi>)
                        n1024 = control-ref of="安装支架线卡扎带安装"() -> (w1301:refnum<vi>)
                        n1025 = for {
                          tunnel: w1325 -> [w1357] mode=indexing
                          i -> [w1356]
                          n1026 = Multiply(x=60, y=w1356) -> (x*y=w1351:i32)
                          n1027 = Add(x=438 ("y"), y=w1351) -> (x+y=w1353:i32)
                          n1028 = Bundle("y"=-1495, w1353) -> (w1352:cluster{"y":i32, i32})  [unwired: 1 in]
                          n1029 = property class="Bool (严格)"(reference=w1357, "Position"=w1352) -> ()  [unwired: 1 in, 2 out]
                        }
                        n1030 = Build Array(w1314, w1313, w1312, w1311, w1310, w1309) -> (w1323:refnum<vi>[])
                        n1031 = control-ref of="安装支架扎带安装"() -> (w1304:refnum<vi>)
                        n1032 = control-ref of="安装扎带和线卡并取走工件"() -> (w1305:refnum<vi>)
                        n1033 = control-ref of="控制器支架安装线卡扎带"() -> ()  [unwired: 1 out]
                        n1034 = control-ref of="控制器支架螺栓5拧紧确认"() -> (w1306:refnum<vi>)
                        n1035 = control-ref of="控制器支架螺栓4拧紧确认"() -> (w1307:refnum<vi>)
                        n1036 = for {
                          tunnel: w1323 -> [w1341] mode=indexing
                          i -> [w1340]
                          n1037 = Multiply(x=60, y=w1340) -> (x*y=w1338:i32)
                          n1038 = Add(x=w1338, y=438) -> (x+y=w1335:i32)
                          n1039 = Bundle("y"=-1145, w1335) -> (w1334:cluster{"y":i32, i32})  [unwired: 1 in]
                          n1040 = property class="Bool (严格)"(reference=w1341, "Position"=w1334) -> ()  [unwired: 1 in, 2 out]
                        }
                        n1041 = Build Array(w1317, w1316, w1315, w1308) -> (w1324:refnum<vi>[])
                        n1042 = Build Array(w1307, w1306, w1305, w1304, w1303, w1302, w1301) -> (w1300:refnum<vi>[])
                        n1043 = for {
                          tunnel: w1324 -> [w1349] mode=indexing
                          i -> [w1348]
                          n1044 = Multiply(x=60, y=w1348) -> (x*y=w1346:i32)
                          n1045 = Add(x=w1346, y=438) -> (x+y=w1343:i32)
                          n1046 = Bundle("y"=-1820, w1343) -> (w1342:cluster{"y":i32, i32})  [unwired: 1 in]
                          n1047 = property class="Bool (严格)"(reference=w1349, "Position"=w1342) -> ()  [unwired: 1 in, 2 out]
                        }
                        n1048 = for {
                          tunnel: w1300 -> [w1333] mode=indexing
                          i -> [w1332]
                          n1049 = Multiply(x=60, y=w1332) -> (x*y=w1330:i32)
                          n1050 = Add(x=w1330, y=438) -> (x+y=w1327:i32)
                          n1051 = Bundle("y"=-100, w1327) -> (w1326:cluster{"y":i32, i32})  [unwired: 1 in]
                          n1052 = property class="Bool (严格)"(reference=w1333, "Position"=w1326) -> ()  [unwired: 1 in, 2 out]
                        }
                      }
                    }
                  }
                  frame Enabled {
                  }
                }
              }
            }
          }
          event "更换产品": Value Change {
            n1053 = event-data() -> ()  [unwired: 1 in, 6 out]
            n1054 = control-ref of="控制器支架安装线卡扎带"() -> (w1387:refnum<vi>)
            n1055 = control-ref of="控制器支架螺栓5拧紧确认"() -> (w1389:refnum<vi>)
            n1056 = control-ref of="控制器支架涂色标"() -> (w1388:refnum<vi>)
            n1057 = control-ref of="控制器支架螺栓3拧紧确认"() -> (w1391:refnum<vi>)
            n1058 = control-ref of="控制器支架螺栓4拧紧确认"() -> (w1390:refnum<vi>)
            n1059 = control-ref of="控制器支架螺栓2拧紧确认"() -> (w1392:refnum<vi>)
            n1060 = control-ref of="控制器支架螺栓1拧紧确认"() -> (w1393:refnum<vi>)
            n1061 = control-ref of="安装支架螺栓4拧紧确认"() -> (w1377:refnum<vi>)
            n1062 = global read "Global.vi" "控制器支架"() -> (w1384:bool[])
            n1063 = control-ref of="安装支架线卡扎带安装"() -> ()  [unwired: 1 out]
            n1064 = control-ref of="安装支架螺栓2拧紧确认"() -> (w1379:refnum<vi>)
            n1065 = control-ref of="安装支架螺栓3拧紧确认"() -> (w1378:refnum<vi>)
            n1066 = control-ref of="安装支架涂色标"() -> (w1376:refnum<vi>)
            n1067 = control-ref of="安装扎带和线卡并取走工件"() -> (w1375:refnum<vi>)
            n1068 = control-ref of="控制器安装螺栓2拧紧确认"() -> (w1382:refnum<vi>)
            n1069 = control-ref of="安装支架螺栓1拧紧确认"() -> (w1380:refnum<vi>)
            n1070 = control-ref of="控制器安装螺栓3拧紧确认"() -> (w1381:refnum<vi>)
            n1071 = control-ref of="控制器安装螺栓1拧紧确认"() -> (w1383:refnum<vi>)
            n1072 = Build Array(w1393, w1392, w1391, w1390, w1389, w1388, w1387) -> (w1363:refnum<vi>[])
            n1073 = for "For循环" {
              tunnel: w1384 -> [w1427] mode=indexing
              tunnel: w1363 -> [w1426] mode=indexing
              shift-right: [w1424] -> _
              shift-left: 360 -> [w1425]
              tunnel: w1363 -> [w1423]
              i -> [w1422]
              n1074 = case shown="真" w1427 {
                tunnel: w1426 -> [w1429 w1431]
                tunnel: w1425 -> [w1430 w1436]
                tunnel: [w1430 w1433] -> w1424
                tunnel: w1423 -> [_ _]
                tunnel: w1422 -> [_ _]
                frame False {
                  n1075 = property class="Bool (严格)"(reference=w1429, "Top"=-100 ("位置:置顶")) -> ()  [unwired: 1 in, 2 out]
                }
                frame True {
                  n1076 = Add(x=w1436, y=50) -> (x+y=w1433:i32)
                  n1077 = Bundle(-1850, w1433) -> (w1434:cluster{i32, i32})  [unwired: 1 in]
                  n1078 = property class="Bool (严格)"(reference=w1431, "Position"=w1434) -> ()  [unwired: 1 in, 2 out]
                }
              }
            }
            n1079 = global read "Global.vi" "控制器安装支架"() -> (w1374:bool[])
            n1080 = Build Array(w1383, w1382, w1381, w1380, w1379, w1378, w1377, w1376, w1375) -> (w1373:refnum<vi>[])
            n1081 = for "For循环" {
              tunnel: w1374 -> [w1412] mode=indexing
              tunnel: w1373 -> [w1411] mode=indexing
              shift-right: [w1409] -> _
              shift-left: 360 -> [w1410]
              tunnel: w1373 -> [w1408]
              n1082 = case shown="真" w1412 {
                tunnel: w1411 -> [w1414 w1416]
                tunnel: w1410 -> [w1415 w1421]
                tunnel: [w1415 w1418] -> w1409
                tunnel: w1408 -> [_ _]
                frame False {
                  n1083 = property class="Bool (严格)"(reference=w1414, "Top"=-100 ("位置:置顶")) -> ()  [unwired: 1 in, 2 out]
                }
                frame True {
                  n1084 = Add(x=w1421, y=50) -> (x+y=w1418:i32)
                  n1085 = Bundle(-1510, w1418) -> (w1419:cluster{i32, i32})  [unwired: 1 in]
                  n1086 = property class="Bool (严格)"(reference=w1416, "Position"=w1419) -> ()  [unwired: 1 in, 2 out]
                }
              }
            }
            n1087 = control-ref of="电机预拧紧螺栓1"() -> (w1370:refnum<vi>)
            n1088 = control-ref of="安装弹性垫圈并按启动拍照"() -> (w1371:refnum<vi>)
            n1089 = control-ref of="请拾取O型圈"() -> (w1362:refnum<vi>)
            n1090 = control-ref of="安装支架扎带安装"() -> ()  [unwired: 1 out]
            n1091 = control-ref of="安装扎带并取走工件"() -> (w1366:refnum<vi>)
            n1092 = control-ref of="请拾取弹簧"() -> (w1361:refnum<vi>)
            n1093 = control-ref of="按启动按钮拍照确认"() -> (w1359:refnum<vi>)
            n1094 = control-ref of="电机安装螺栓2扭矩确认"() -> (w1360:refnum<vi>)
            n1095 = control-ref of="电机安装螺栓1扭矩确认"() -> (w1368:refnum<vi>)
            n1096 = control-ref of="涂色标"() -> (w1367:refnum<vi>)
            n1097 = control-ref of="电机预拧紧螺栓2"() -> (w1369:refnum<vi>)
            n1098 = global read "Global.vi" "电机安装"() -> (w1365:bool[])
            n1099 = Build Array(w1361, w1362, w1371, w1370, w1369, w1368, w1360, w1359, w1367, w1366) -> (w1358:refnum<vi>[])
            n1100 = for "For循环" {
              tunnel: w1365 -> [w1398] mode=indexing
              tunnel: w1358 -> [w1397] mode=indexing
              shift-right: [w1395] -> _
              shift-left: 360 -> [w1396]
              tunnel: w1358 -> [w1394]
              n1101 = case shown="真" w1398 {
                tunnel: w1397 -> [w1400 w1402]
                tunnel: w1396 -> [w1401 w1407]
                tunnel: [w1401 w1404] -> w1395
                tunnel: w1394 -> [_ _]
                frame False {
                  n1102 = property class="Bool (严格)"(reference=w1400, "Top"=-100 ("位置:置顶")) -> ()  [unwired: 1 in, 2 out]
                }
                frame True {
                  n1103 = Add(x=w1407, y=50) -> (x+y=w1404:i32)
                  n1104 = Bundle(-1193, w1404) -> (w1405:cluster{i32, i32})  [unwired: 1 in]
                  n1105 = property class="Bool (严格)"(reference=w1402, "Position"=w1405) -> ()  [unwired: 1 in, 2 out]
                }
              }
            }
            n1106 = global write "A170316-11.vi" "电机安装LED"(w1358) -> ()
            "产品型号" <- w1385
          }
          event Panel Close {
            n1107 = event-data() -> ()  [unwired: 1 in, 4 out]
            n1108 = global write "Global.vi" "程序关闭"(TRUE ("程序关闭")) -> ()
          }
        }
        n1109 = case shown="真" w1080 {
          tunnel: w1079 -> [_ w1082]
          frame False {
          }
          frame True {
            n1110 = property on="更换布局" class="Str"("Val(Sgnl)"=w1082) -> ()  [unwired: 2 in, 2 out]
          }
        }
        n1111 = control-ref of="更换产品"() -> (w1077:refnum<vi>)
        n1112 = global write "Global.vi" "更换产品"(w1077) -> ()
        n1113 = global read "Global.vi" "程序关闭"() -> (w1078:bool)
      }
    }
  }
